vi "main.vi"(0 "Test Pins":T13, 1 "Caller Information":T10, 5 "Test Inputs":T7={"Load Current in A"=0.0, "Frequency in Hz"=[], "Input Voltage in V"=0.0, "FGen Peak-Peak Voltage in V"=1.0, "Resolution bandwidth in %"=1.0, "Sampling Rate multiplier"=10.0, "Take PSRR snapshot?"=TRUE, "Acquisition Time(s)"=0.2, "Horizontal Timing"=enum."Calculate Sampling Rate", "Advance Setting"={"Prepare"={"Load SMU Output Function"=enum."VoltageSource"}, "Stimulus and Measure"={"Loop Delay"=1, "Autoset Sampling Rate?"=TRUE, "Search Tolerance (+/- % of Freq.)"=5.0}}}, 11 "error in":errorcluster) -> (4 "Test Results":T14 {"Record Length in S" format="%#.5g"; "Sample Rate in S/s" format="%#.5g"; "PSRR in dB" format="%#.5g"; "Frequency in Hz" format="%#.5g"; "Detected Vin_ac_pp in V" format="%#.5g"; "Detected Vout_ac_pp in V" format="%#.5g"}, 15 "error out":errorcluster)   [LabVIEW 2020, in "LDO PSRR.lvlib"]
doc: "<b>Caller</b> Information is input for framework components. Mode should be set to <b>Automation</b> when running from TestStand. Sequence Context should be set to <b>ThisContext</b> when running from TestStand. The values will be updated everytime the setting is applied using \"Edit\" dialog.\n\n<b>Test Pins</b> is names of pins available in the pinmap file. Provide the right pins for the required functionality.\n\n<b>Test Inputs</b> is input required for the measurement to perform.\n\n<b>error in</b> is meant for the sequencing. <b>error in</b> should be <b>no error</b> always.\n\n<b>Test Results</b> contains all the measured data during the measurement and processed results.\n\n<b>error out</b> contains the error occured during measurement.\n\nCheck measurement documentation for more information (<Program Files>\\Soliton Technologies\\MeasurementSuite\\CodeModules\\LDO\\LDO PSRR.pdf)"
uses:
  LDO PSRR.lvlib
  Typedefs/Test Results.ctl
  Typedefs/Test Inputs.ctl
  Typedefs/Advance Test Input.ctl
  Reusables/Instrument APIs/Load Output Function.ctl
  <userlib>/_Soliton/Measurement Suite/Reusables/Plugin Common/Typedefs/Caller Events.ctl
  <userlib>/_Soliton/Measurement Suite/Reusables/Plugin Common/Typedefs/Caller Information.ctl
  <userlib>/_Soliton/Measurement Suite/Reusables/Plugin Common/Typedefs/Caller Mode.ctl
  Typedefs/Test Pins.ctl
  Typedefs/Pin Dropdown.ctl
  <userlib>/_Soliton/Measurement Suite/Reusables/Plugin Common/Typedefs/Termination Monitor Info.ctl
  <instrlib>/niFgen/niFgen.llb/niFgen Output Mode.ctl
  <instrlib>/niFgen/niFgen.llb/niFgen Waveform Type.ctl
  <vilib>/Utility/error.llb/DialogType.ctl
  ed717c1b-eec1-43b4-99c1-3d83852bef44.vi
  00c9e72c-dc14-40c2-acfc-7b2698a37ca7.vi
  d9360132-6dee-4b9e-876e-39170c807331.vi
  f5d431a0-41a8-4d91-8ed4-f3030fcb2f72.vi
  e32b1f2d-d2d3-47cf-a8ae-c4d1a59e525c.vi
  bb3e62c4-a2c2-4505-9438-f842dd651d6c.vi
  ce2ee1e5-697c-4608-b941-8c9b0f21ffd9.vi
  9f6bafd6-9b9c-4545-a9d9-e38da2077c76.vi
  c4032409-4502-45fd-bca3-2506d9579697.vi
  b2eee2bd-4b89-4e54-a034-5f4da275eb34.vi
  <userlib>/_Soliton/Measurement Suite/Reusables/InstrumentSessionAPIs/SessionManagerApiPath.vi
  <vilib>/Utility/sysdir.llb/Get System Directory.vi
  <vilib>/Utility/LVLibp/Get Exported File Path.vi
  <userlib>/_Soliton/Measurement Suite/Reusables/Errors/Error 6001.vi
  <userlib>/_Soliton/Measurement Suite/Reusables/Plugin Common/Plugin Common.lvlib
  <userlib>/_Soliton/Measurement Suite/Reusables/Queue Driver/Plugin Queue Driver.lvlib
panel:
  out "Progress":i32(slide) scale=-1.0..5.0
  in  "Terminate":bool
  in  "Run":bool caption="Measure"
  in  "Exit":bool
  out "Header":string
  in  "Tab Enum":T1(radio)
  out "Tab Control":T2(tab)
  in  "SystemSetup":T4={"Set Input Voltage"={"PinStatus"=0, "PinName"="", "Info"=TRUE}, "Set Frequency"={"PinStatus"=0, "PinName"="", "Info"=TRUE}, "Set Load Current"={"PinStatus"=0, "PinName"="", "Info"=TRUE}, "Measure Input Voltage"={"PinStatus"=0, "PinName"="", "Info"=TRUE}, "Measure Output Voltage"={"PinStatus"=0, "PinName"="", "Info"=TRUE}}
  in  "Sampling Rate Multiplier":dbl=10.0 min=2.0 max=100.0 format="%#_6p"
  in  "Minimum Resolution Bandwidth (%)":dbl=1.0 min=0.001 max=100.0 format="%#_6f"
  in  "Step Input":T5={"Minimum Frequency (Hz)"=10.0, "Maximum Frequency (Hz)"=10000000.0} {"Maximum Frequency (Hz)" min=10.0 max=80000000.0 format="%#_6p"; "Minimum Frequency (Hz)" items=["10Hz"=10.0, "100Hz"=100.0, "1kHz"=1000.0, "100kHz"=100000.0]}
  in  "Customize Sweep Value":bool
  in  "Input Voltage (V)":dbl format="%#_6p"
  in  "Load Current (A)":dbl format="%#_6p"
  in  "Advanced Settings":bool
  in  "Pk-Pk Voltage (V)":dbl=1.0 caption="FGen Peak-Peak Voltage (V)" format="%#_6p"
  in  "Frequency (Hz)":dbl[](array[numeric]) format="%#_6p"
  out "Result Tab":T6(tab)
  out "Frequency Vs PSRR":cluster{"Iload (mA)":dbl[], "Vout (V)":dbl[]}(graph)
  in  "Take PSRR snapshot?":bool=TRUE
  out "Measured Values":string[][](table)
  in  "Result Enum":T6(radio)
  in  "ErrorOccured":errorcluster
  in  "Caller Events":T12
  in  "DataLogPath":path
  # "Supports NIScopeInstrument"
  # "Supports NIScopeInstrument"
  # "Supports NIFGenInstrument"
  # "Supports NIDCPowerInstrument"
  # "Supports NIDCPowerInstrument"
  # "SMU Settings"
  # "FGen Settings"
  # "Fill Frequency using the following"
  # "Oscilloscope Settings"
  # "Resolution Bandwidth (%) is the percentage of minimum separation required between two frequency\nMinimum Sampling Rate = Frequency * Sampling Rate Multiplier"
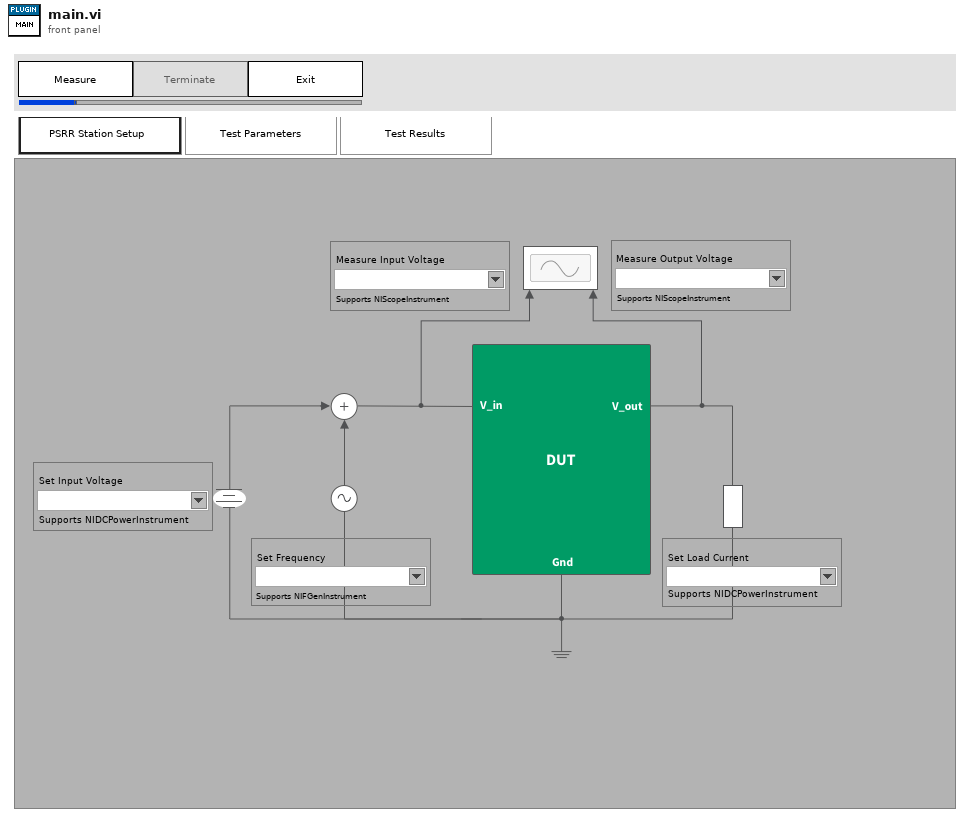
[diagram p1: front panel]
types:
  T1 = enum32{"Station Setup", "Test Parameters", "Test Results"}
  T2 = enum32{"Station Setup", "Test Parameters", "Test Results", "Debug"}
  T3 = typedef "LDO PSRR.lvlib/Pin Dropdown.ctl" = cluster{"PinStatus":u16, "PinName":string, "Info":bool}
  T4 = cluster{"Set Input Voltage":T3, "Set Frequency":T3, "Set Load Current":T3, "Measure Input Voltage":T3, "Measure Output Voltage":T3}
  T5 = cluster{"Minimum Frequency (Hz)":dbl, "Maximum Frequency (Hz)":dbl}
  T6 = enum32{"Line Regulation Curve", "Measured Value Table View"}
  T7 = typedef "LDO PSRR.lvlib/Test Inputs.ctl" = cluster{"Load Current in A":dbl, "Frequency in Hz":dbl[], "Input Voltage in V":dbl, "FGen Peak-Peak Voltage in V":dbl, "Resolution bandwidth in %":dbl, "Sampling Rate multiplier":dbl, "Take PSRR snapshot?":bool, "Acquisition Time(s)":dbl, "Horizontal Timing":enum32{"Calculate Sampling Rate", "Calculate Acquisition Time", "Calculate Record Length"}, "Advance Setting":T8}
  T8 = typedef "LDO PSRR.lvlib/Advance Test Input.ctl" = cluster{"Prepare":cluster{"Load SMU Output Function":T9}, "Stimulus and Measure":cluster{"Loop Delay":u32, "Autoset Sampling Rate?":bool, "Search Tolerance (+/- % of Freq.)":dbl}}
  T9 = typedef "Load Output Function.ctl" = enum16{"VoltageSource", "CurrentSource"}
  T10 = typedef "Plugin Common.lvlib/Caller Information.ctl" = cluster{"Mode":T11, "Sequence Context":refnum<k7>}
  T11 = typedef "Plugin Common.lvlib/Caller Mode.ctl" = enum16{"Standalone", "Automation", "MeasurementSuite"}
  T12 = typedef "Plugin Common.lvlib/Caller Events.ctl" = cluster{"Caller Event":refnum<user-event>}
  T13 = typedef "LDO PSRR.lvlib/Test Pins.ctl" = cluster{"Set Input Voltage":string, "Measure Input Voltage":string, "Set Load Current":string, "Measure Output Voltage":string, "Set Frequency":string}
  T14 = typedef "LDO PSRR.lvlib/Test Results.ctl" = cluster{"Frequency in Hz":dbl[], "Detected Vin_ac_pp in V":dbl[], "Detected Vout_ac_pp in V":dbl[], "PSRR in dB":dbl[], "Sample Rate in S/s":dbl[], "Record Length in S":dbl[]}
  T15 = typedef "Plugin Common.lvlib/Termination Monitor Info.ctl" = cluster{"Caller Information":T10, "Execution":refnum<k7>, "Termination Monitor":refnum<k7>, "Type":string, "Plugin Name":string}
  T16 = cluster{"Termination Monitor Info":T15, "Test Inputs":T7, "Test Results":T14, "Test Results[][]":string[][], "Test Pins":T13, "Logger Folder Path":path, "Scope Channels":string, "Valid Logger path?":bool, "Logger file path":path, "UI Ctls":refnum<vi>[], "Minimum Sampling Rate (S/s)":dbl, "Minimum Record Length (S)":i32}
  T17 = enum8{"Enabled", "Disabled", "Disabled and Grayed Out"}
  T18 = cluster{"Set Vin":T3, "Set Frequency":T3, "Set Iload":T3, "Measure Vin":T3, "Measure Vout":T3}
  T19 = cluster{"Minimum Frequency (Hz)":dbl, "Maximum Frequency Hz)":dbl}
  T20 = typedef "niFgen Waveform Type.ctl" = i32
  T21 = typedef "niFgen Output Mode.ctl" = u32
  T22 = cluster{"relativeInitialX":dbl, "xIncrement":dbl, "wfm":dbl[]}
  T23 = cluster{"Frequency in Hz":dbl[], "PSRR in dB":dbl[]}
  T24 = typedef "DialogType.ctl" = u16
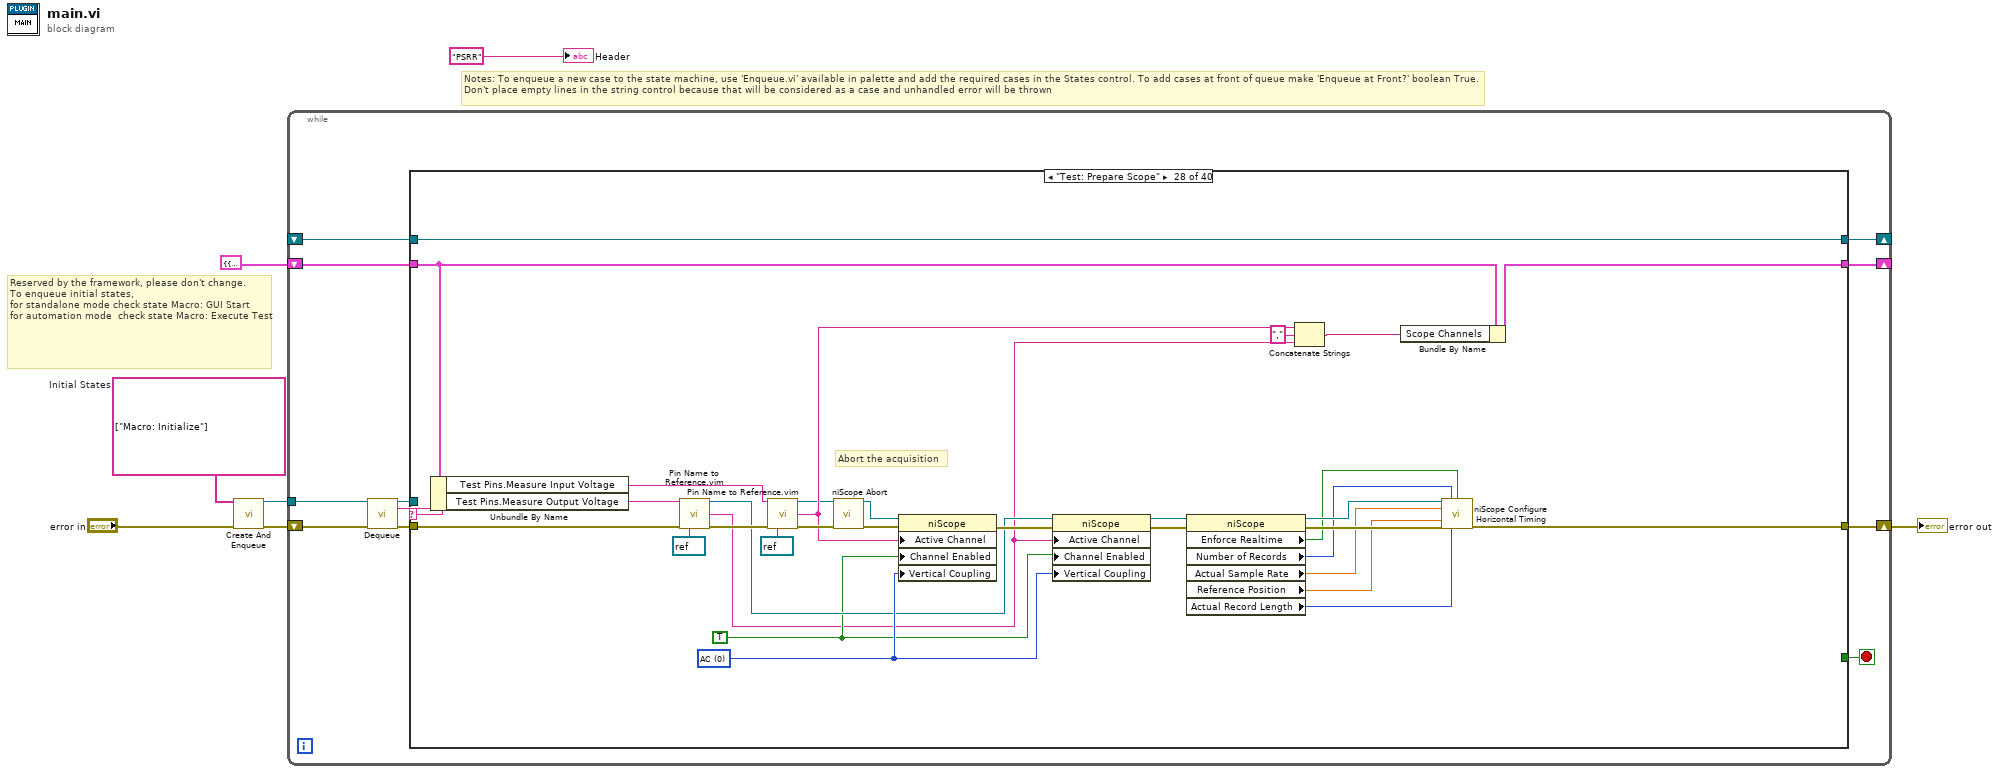
[diagram p0: block diagram]
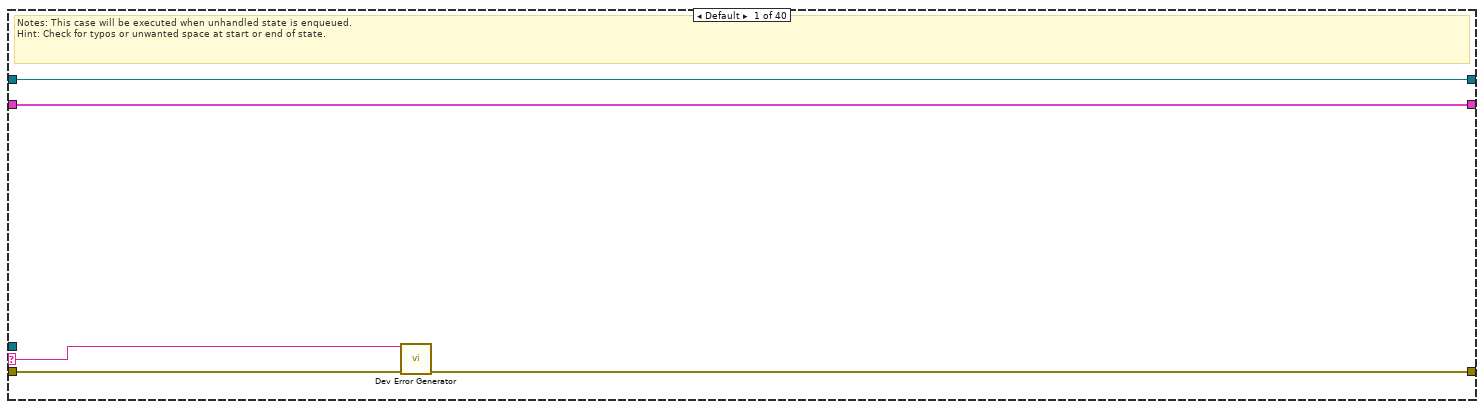
[diagram p2: hidden frame]
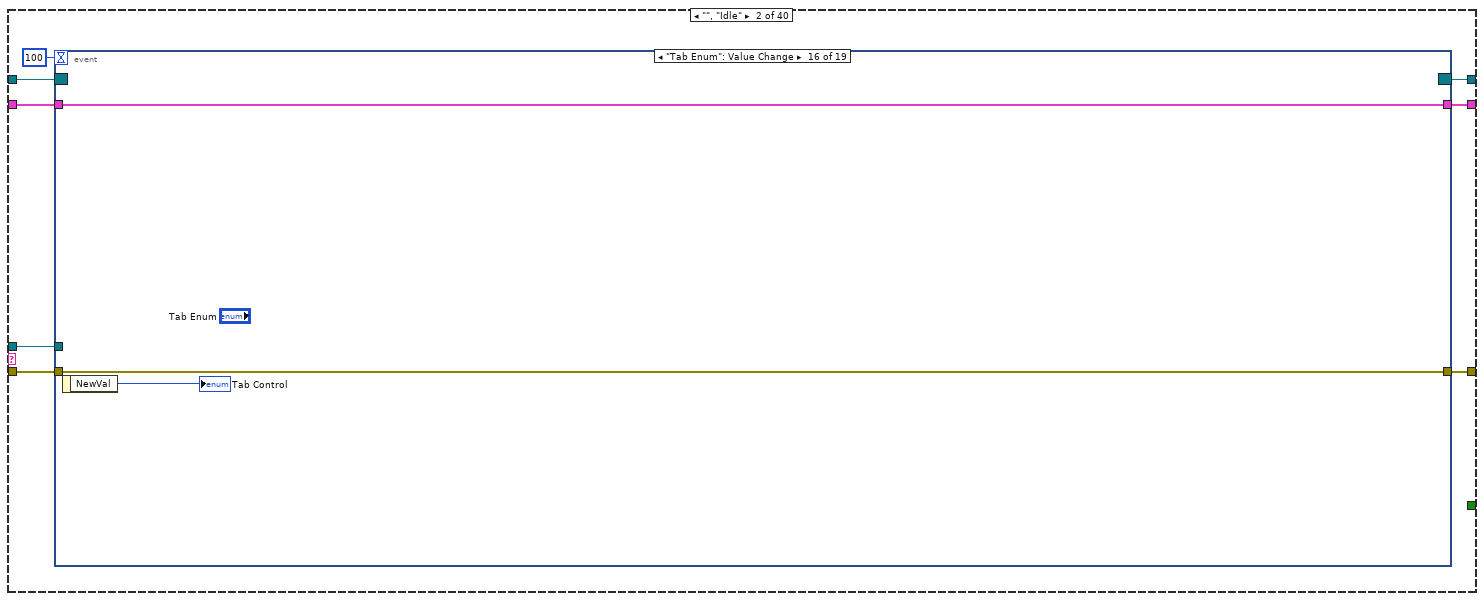
[diagram p3: hidden frame]
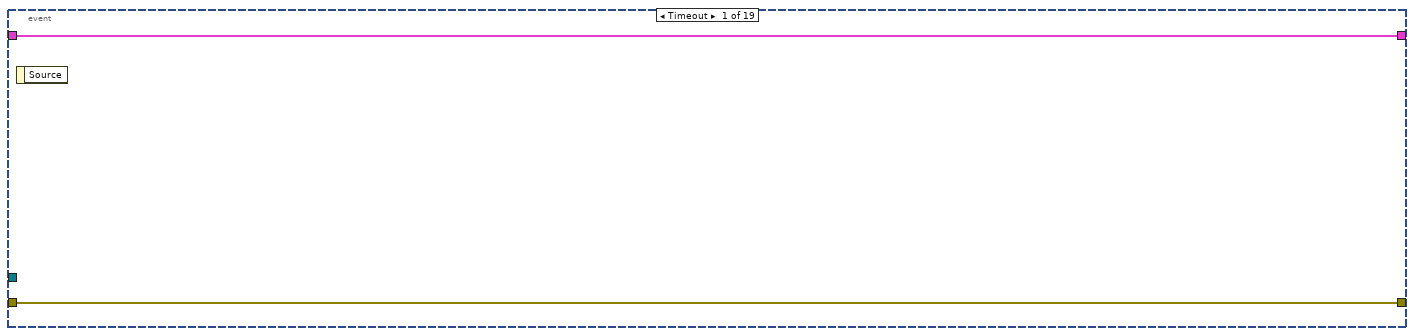
[diagram p4: hidden frame]
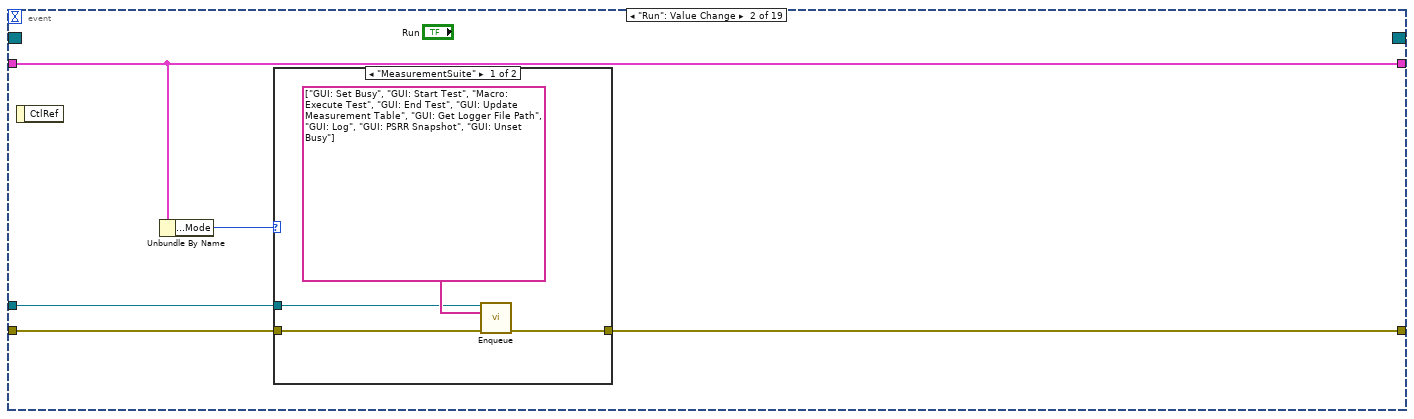
[diagram p5: hidden frame]
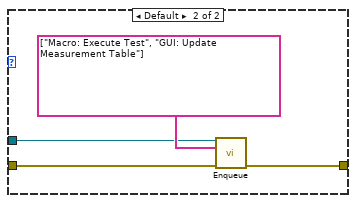
[diagram p6: hidden frame]
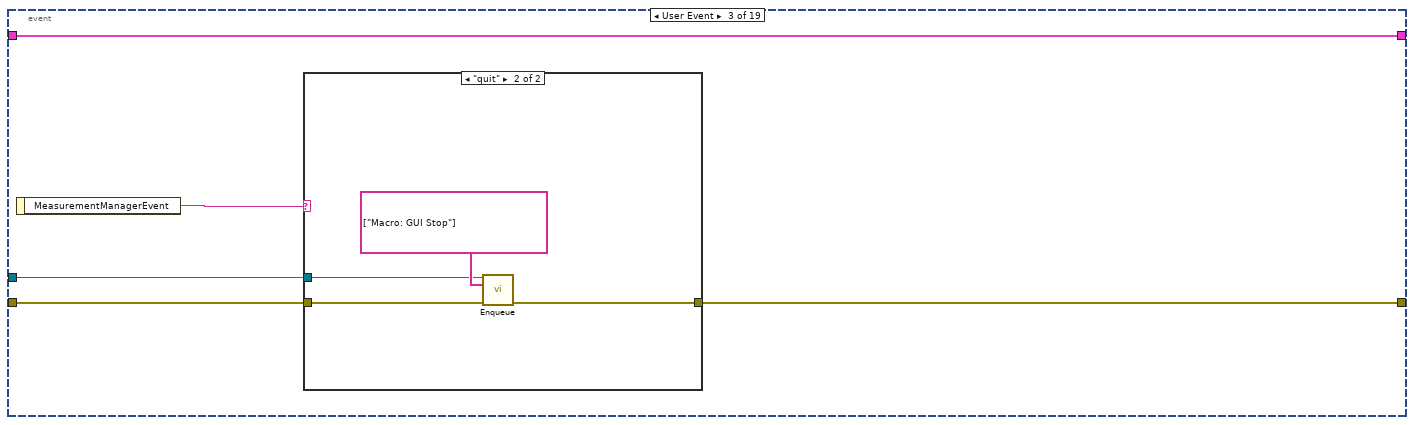
[diagram p7: hidden frame]
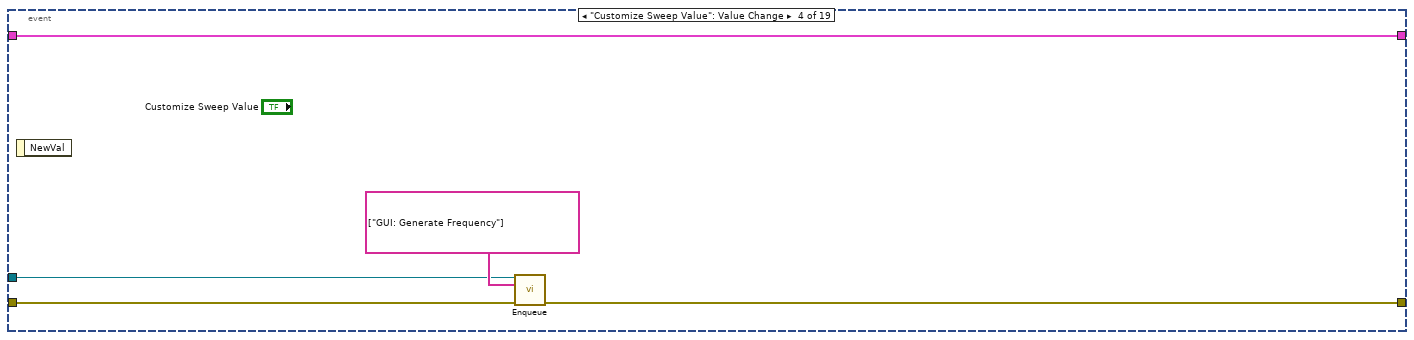
[diagram p9: hidden frame]
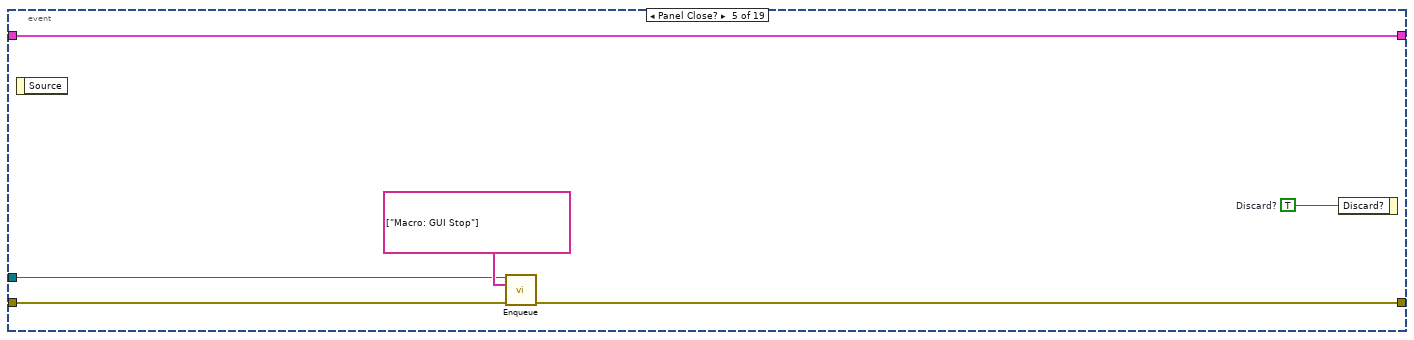
[diagram p10: hidden frame]
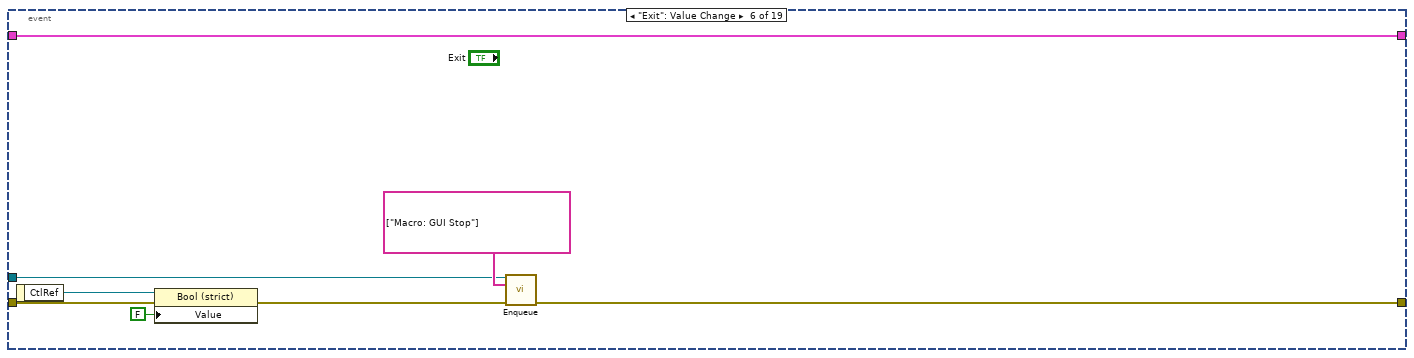
[diagram p11: hidden frame]
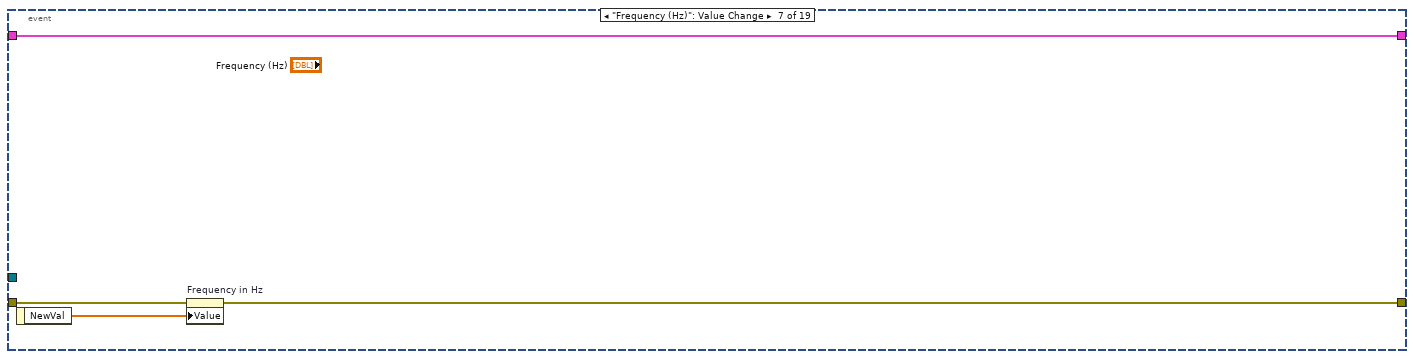
[diagram p12: hidden frame]
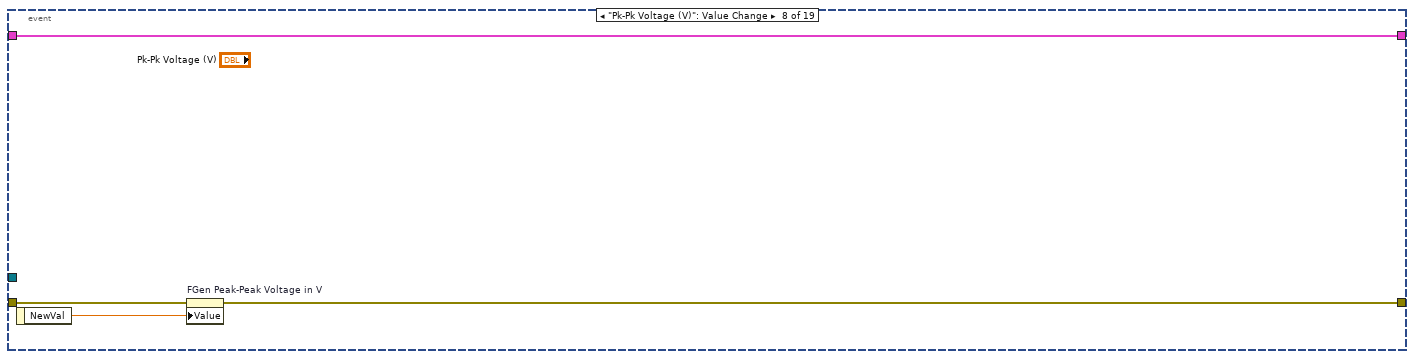
[diagram p13: hidden frame]
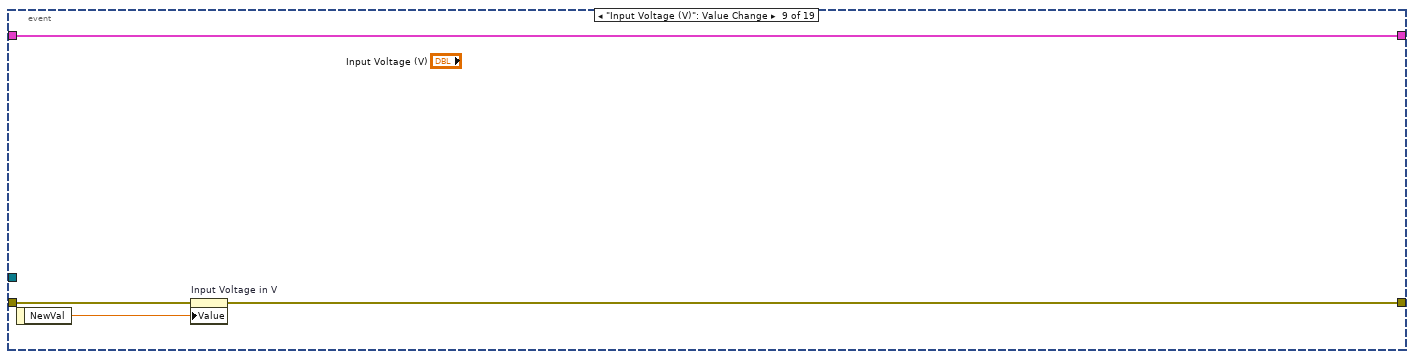
[diagram p14: hidden frame]
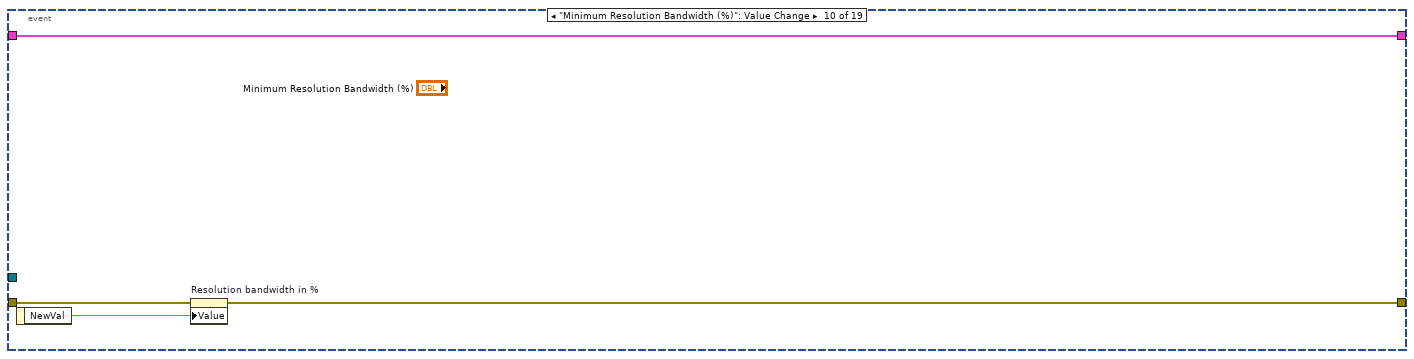
[diagram p15: hidden frame]
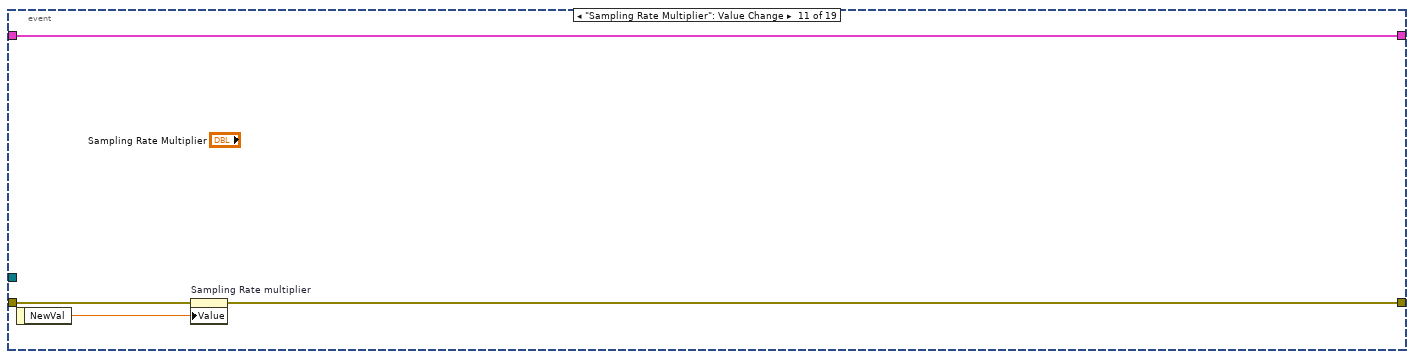
[diagram p16: hidden frame]
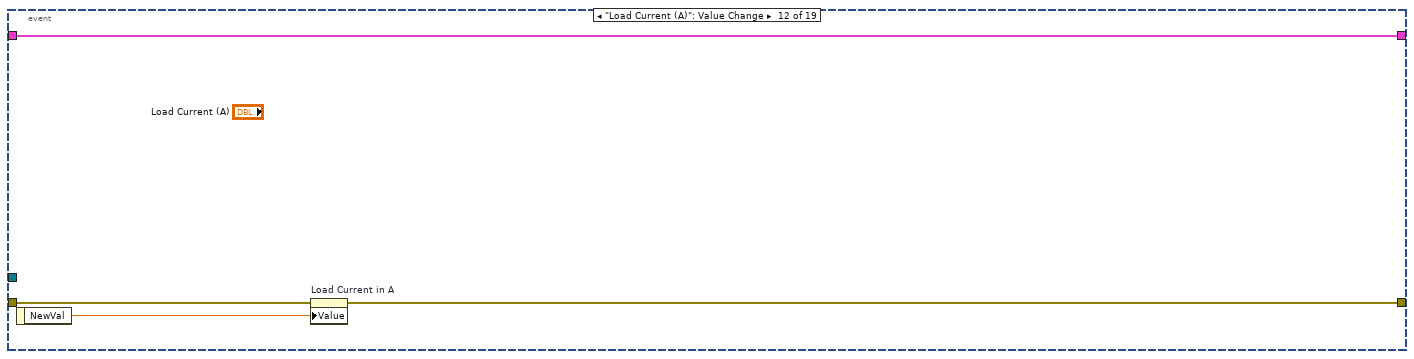
[diagram p17: hidden frame]
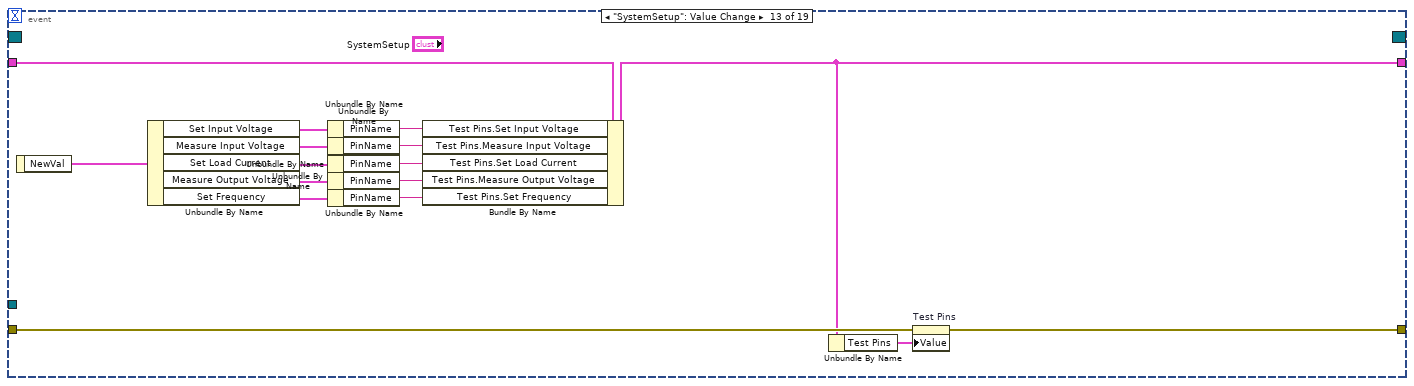
[diagram p18: hidden frame]
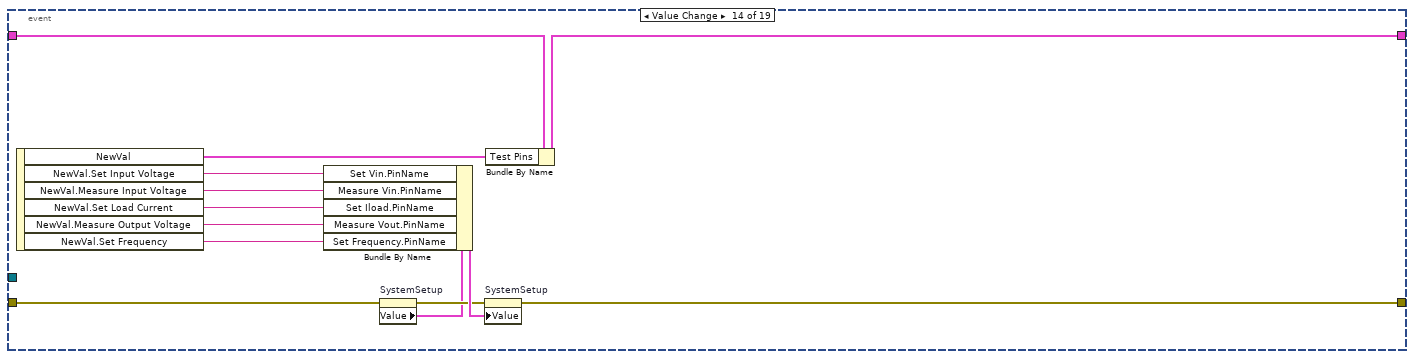
[diagram p19: hidden frame]
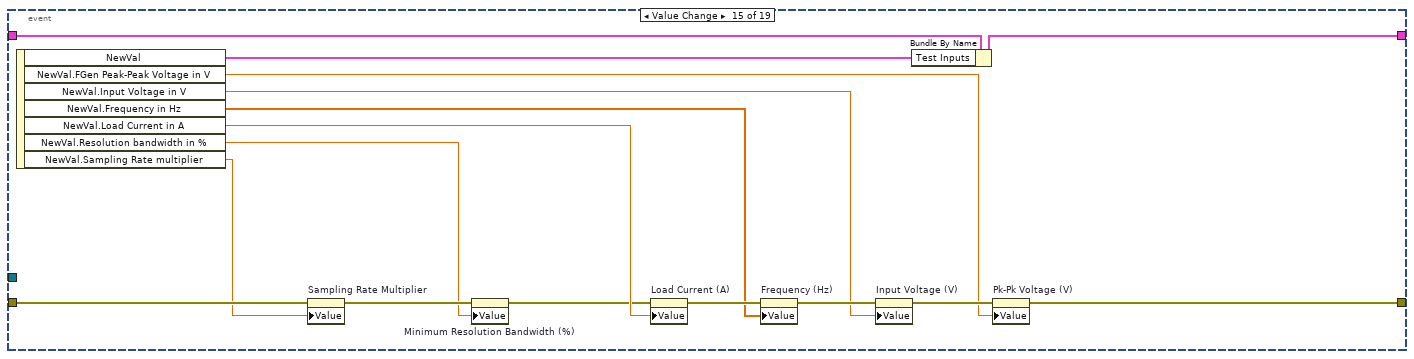
[diagram p20: hidden frame]
diagram:
  w7 = string[] ["Macro: Initialize"]  # Initial States
  # "Notes: To enqueue a new case to the state machine, use 'Enqueue.vi' available in palette and add the required cases in the States control. To add cases at front of queue make 'Enqueue at Front?' boolean True. Don't place empty lines in the string control because that will be considered as a case and unhandled error will be thrown"
  # "Reserved by the framework, please don't change. \nTo enqueue initial states,\nfor standalone mode check state Macro: GUI Start\nfor automation mode  check state Macro: Execute Test"
  n1 = call <userlib>:"Create And Enqueue.vi"("Initial States"=w7, "error in (no error)"="error in") -> ("Queue out"=w5:refnum<queue>, "error out"=w3:errorcluster)  [unwired: 12 in]
  n2 = while {
    shift-right: [w18] -> w4
    shift-left: w3 -> [w16]
    shift-right: [w14] -> _
    shift-left: T16 {"Termination Monitor Info"={"Caller Information"={"Mode"=enum."Standalone", "Sequence Context"=refnum}, "Execution"=refnum, "Termination Monitor"=refnum, "Type"="", "Plugin Name"=""}, "Test Inputs"={"Load Current in A"=0.0, "Frequency in Hz"=[], "Input Voltage in V"=0.0, "FGen Peak-Peak Voltage in V"=0.0, "Resolution bandwidth in %"=20000000.0, "Sampling Rate multiplier"=1000.0, "Take PSRR snapshot?"=FALSE, "Acquisition Time(s)"=0.0, "Horizontal Timing"=enum."Calculate Sampling Rate", "Advance Setting"={"Prepare"={"Load SMU Output Function"=enum."VoltageSource"}, "Stimulus and Measure"={"Loop Delay"=0, "Autoset Sampling Rate?"=TRUE, "Search Tolerance (+/- % of Freq.)"=0.0}}}, "Test Results"={"Frequency in Hz"=[], "Detected Vin_ac_pp in V"=[], "Detected Vout_ac_pp in V"=[], "PSRR in dB"=[], "Sample Rate in S/s"=[], "Record Length in S"=[]}, "Test Results[][]"=[], "Test Pins"={"Set Input Voltage"="", "Measure Input Voltage"="", "Set Load Current"="", "Measure Output Voltage"="", "Set Frequency"=""}, "Logger Folder Path"=path "", "Scope Channels"="", "Valid Logger path?"=FALSE, "Logger file path"=path "", "UI Ctls"=[], "Minimum Sampling Rate (S/s)"=0.0, "Minimum Record Length (S)"=0} -> [w13]
    tunnel: w5 -> [w12]
    shift-right: [w9] -> _
    shift-left: _ -> [w10]
    stop <- w17 stop-if-true
    n3 = call <userlib>:"Dequeue.vi"("Queue in"=w12, "error in (no error)"=w16) -> ("Queue out"=w11:refnum<queue>, "Dequeued State"=w8:string, "error out"=w15:errorcluster)  [unwired: 11 in]
    n4 = case shown="\"Test: Prepare Scope\"" w8 {
      selector: w8 -> [w21 _ _ _ _ _ _ _ _ _ _ _ _ _ _ _ _ _ _ _ _ _ _ _ _ _ _ _ _ _ _ _ _ _ _ _ _ _ _ _]
      tunnel: w15 -> [w20 w28 w164 w173 w182 w189 w196 w201 w228 w239 w243 w246 w257 w272 w277 w290 w306 w321 w345 w359 w376 w386 w391 w398 w403 w417 w427 w459 w466 w473 w497 w595 w606 w624 w636 w638 w650 w658 w665 w683]
      tunnel: [w22 w29 w164 w176 w183 w190 w197 w201 w226 w237 w241 w246 w251 w272 w276 w289 w307 w319 w346 w360 w377 w386 w392 w399 w403 w411 w424 w458 w464 w471 w499 w580 w599 w612 w636 w638 w647 w658 w663 w677] -> w18
      tunnel: [_ _ _ _ _ _ _ _ _ _ _ _ _ _ _ _ _ _ _ _ _ _ _ _ _ _ _ _ _ _ _ _ _ _ _ _ _ _ w660 TRUE] -> w17
      tunnel: [w23 w31 w163 w166 w184 w191 w198 w200 w217 w238 w242 w245 w249 w266 w278 w291 w304 w316 w347 w361 w383 w385 w390 w397 w402 w410 w429 w457 w465 w472 w501 w597 w608 w626 w635 w644 w655 w657 w662 w684] -> w14
      tunnel: w13 -> [w23 w30 w163 w177 w184 w191 w198 w200 w233 w238 w242 w245 w248 w265 w278 w291 w304 w315 w347 w361 w383 w385 w389 w396 w402 w420 w429 w456 w465 w472 w502 w597 w608 w626 w634 w644 w655 w657 w662 w684]
      tunnel: w11 -> [_ w24 _ w175 w180 w187 w194 _ _ _ _ _ _ _ _ _ _ _ _ _ _ _ _ _ _ _ _ _ _ _ _ _ _ _ _ _ _ _ w659 w682]
      tunnel: w10 -> [w19 w26 w162 w174 w179 w186 w193 w199 w232 _ w240 w244 w258 w271 w284 w297 w313 w322 w348 w362 w382 w384 w393 w400 w401 w419 w430 w461 w467 w474 w500 w598 w609 w627 w637 w643 w654 w656 w664 w681]
      tunnel: [w19 w25 w162 w174 w179 w186 w193 w199 w232 w236 w240 w244 w258 w271 w284 w297 w313 w322 w348 w362 w382 w384 w393 w400 w401 w419 w430 w461 w467 w474 w500 w598 w609 w627 w637 w643 w654 w656 w664 w681] -> w9
      frame Default {
        # "Notes: This case will be executed when unhandled state is enqueued. \nHint: Check for typos or unwanted space at start or end of state."
        n5 = call <userlib>:"Dev Error Generator.vi"("State"=w21, "error in (no error)"=w20) -> ("error out"=w22:errorcluster)  [unwired: 13 in]
      }
      frame "", "Idle" {
        n6 = event shown="[15] \"Tab Enum\": Value Change" {
          selector: w26 -> [_ _ _ _ _ _ _ _ _ _ _ _ _ _ _ _ _ _ _]
          dyn-events: [_ _ _ _ _ _ _ _ _ _ _ _ _ _ _ _ _ _ _] -> w25
          timeout: 100 -> [_ _ _ _ _ _ _ _ _ _ _ _ _ _ _ _ _ _ _]
          tunnel: [w33 w35 w51 w61 w67 w75 w76 w81 w87 w91 w95 w99 w101 w126 w140 w147 w150 w154 w160] -> w31
          tunnel: w30 -> [w33 w35 w51 w61 w67 w75 w76 w81 w87 w91 w95 w99 w105 w125 w139 w147 w150 w154 w159]
          tunnel: [w32 w38 w49 w59 w64 w73 w78 w82 w86 w90 w94 w98 w103 w127 w142 w146 w149 w152 w156] -> w29
          tunnel: w28 -> [w32 w37 w50 w58 w63 w72 w79 w83 w85 w89 w93 w97 w102 w128 w133 w146 w149 w153 w161]
          tunnel: w24 -> [_ w36 w47 w57 w62 w71 _ _ _ _ _ _ _ _ _ _ _ _ _]
          event Timeout {
            n7 = event-data() -> ()  [unwired: 1 in, 1 out]
          }
          event "Run": Value Change {
            n8 = event-data() -> ()  [unwired: 1 in, 1 out]
            n9 = Unbundle By Name(w35) -> ("Termination Monitor Info.Caller Information.Mode"=w34:T11)
            n10 = case shown="\"MeasurementSuite\"" w34 {
              tunnel: [w41 w45] -> w38
              tunnel: w37 -> [w40 w44]
              tunnel: w36 -> [w39 w43]
              frame "MeasurementSuite" {
                n11 = call <userlib>:"Enqueue.vi"("Queue in"=w39, "States"=string[] ["GUI: Set Busy", "GUI: Start Test", "Macro: Execute Test", "GUI: End Test", "GUI: Update Measurement Table", "GUI: Get Logger File Path", "GUI: Log", "GUI: PSRR Snapshot", "GUI: Unset Busy"], "error in (no error)"=w40) -> ("error out"=w41:errorcluster)  [unwired: 11 in, 1 out]
              }
              frame Default {
                n12 = call <userlib>:"Enqueue.vi"("Queue in"=w43, "States"=string[] ["Macro: Execute Test", "GUI: Update Measurement Table"], "error in (no error)"=w44) -> ("error out"=w45:errorcluster)  [unwired: 11 in, 1 out]
              }
            }
          }
          event User Event {
            n13 = event-data() -> ("MeasurementManagerEvent"=w48:string)  [unwired: 1 in]
            n14 = case shown="\"quit\"" w48 {
              tunnel: [w52 w53] -> w49
              tunnel: w50 -> [w52 w55]
              tunnel: w47 -> [_ w54]
              frame Default {
              }
              frame "quit" {
                n15 = call <userlib>:"Enqueue.vi"("Queue in"=w54, "States"=string[] ["Macro: GUI Stop"], "error in (no error)"=w55) -> ("error out"=w53:errorcluster)  [unwired: 11 in, 1 out]
              }
            }
          }
          event "Customize Sweep Value": Value Change {
            n16 = event-data() -> ()  [unwired: 1 in, 1 out]
            n17 = call <userlib>:"Enqueue.vi"("Queue in"=w57, "States"=string[] ["GUI: Generate Frequency"], "error in (no error)"=w58) -> ("error out"=w59:errorcluster)  [unwired: 11 in, 1 out]
          }
          event Panel Close? {
            w66 = TRUE  # Discard?
            n18 = event-data() -> ()  [unwired: 1 in, 1 out]
            n19 = call <userlib>:"Enqueue.vi"("Queue in"=w62, "States"=string[] ["Macro: GUI Stop"], "error in (no error)"=w63) -> ("error out"=w64:errorcluster)  [unwired: 11 in, 1 out]
            n20 = event-data("Discard?"=w66) -> ()  [unwired: 1 in, 1 out]
          }
          event "Exit": Value Change {
            n21 = event-data() -> ("CtlRef"=w69:refnum<vi>)  [unwired: 1 in]
            n22 = property class="Bool (strict)"(reference=w69, error in=w72, "Value"=FALSE) -> (error out=w70:errorcluster)  [unwired: 1 out]
            n23 = call <userlib>:"Enqueue.vi"("Queue in"=w71, "States"=string[] ["Macro: GUI Stop"], "error in (no error)"=w70) -> ("error out"=w73:errorcluster)  [unwired: 11 in, 1 out]
          }
          event "Frequency (Hz)": Value Change {
            n24 = event-data() -> ("NewVal"=w77:dbl[])  [unwired: 1 in]
            n25 = property on="Frequency in Hz" class="Arr (strict)"(error in=w79, "Value"=w77) -> (error out=w78:errorcluster)  [unwired: 1 in, 1 out]
          }
          event "Pk-Pk Voltage (V)": Value Change {
            n26 = event-data() -> ("NewVal"=w80:dbl)  [unwired: 1 in]
            n27 = property on="FGen Peak-Peak Voltage in V" class="DigNum (strict)"(error in=w83, "Value"=w80) -> (error out=w82:errorcluster)  [unwired: 1 in, 1 out]
          }
          event "Input Voltage (V)": Value Change {
            n28 = event-data() -> ("NewVal"=w84:dbl)  [unwired: 1 in]
            n29 = property on="Input Voltage in V" class="DigNum (strict)"(error in=w85, "Value"=w84) -> (error out=w86:errorcluster)  [unwired: 1 in, 1 out]
          }
          event "Minimum Resolution Bandwidth (%)": Value Change {
            n30 = event-data() -> ("NewVal"=w88:dbl)  [unwired: 1 in]
            n31 = property on="Resolution bandwidth in %" class="DigNum (strict)"(error in=w89, "Value"=w88) -> (error out=w90:errorcluster)  [unwired: 1 in, 1 out]
          }
          event "Sampling Rate Multiplier": Value Change {
            n32 = event-data() -> ("NewVal"=w92:dbl)  [unwired: 1 in]
            n33 = property on="Sampling Rate multiplier" class="DigNum (strict)"(error in=w93, "Value"=w92) -> (error out=w94:errorcluster)  [unwired: 1 in, 1 out]
          }
          event "Load Current (A)": Value Change {
            n34 = event-data() -> ("NewVal"=w96:dbl)  [unwired: 1 in]
            n35 = property on="Load Current in A" class="DigNum (strict)"(error in=w97, "Value"=w96) -> (error out=w98:errorcluster)  [unwired: 1 in, 1 out]
          }
          event "SystemSetup": Value Change {
            n36 = event-data() -> ("NewVal"=w104:T4)  [unwired: 1 in]
            n37 = Unbundle By Name(w104) -> ("Set Input Voltage"=w110:T3, "Measure Input Voltage"=w109:T3, "Set Load Current"=w108:T3, "Measure Output Voltage"=w107:T3, "Set Frequency"=w106:T3)
            n38 = Unbundle By Name(w110) -> ("PinName"=w115:string)
            n39 = Unbundle By Name(w109) -> ("PinName"=w114:string)
            n40 = Unbundle By Name(w108) -> ("PinName"=w113:string)
            n41 = Unbundle By Name(w107) -> ("PinName"=w112:string)
            n42 = Unbundle By Name(w106) -> ("PinName"=w111:string)
            n43 = Bundle By Name(cluster=w105, "Test Pins.Set Input Voltage"=w115, "Test Pins.Measure Input Voltage"=w114, "Test Pins.Set Load Current"=w113, "Test Pins.Measure Output Voltage"=w112, "Test Pins.Set Frequency"=w111) -> (w101:T16)
            n44 = Unbundle By Name(w101) -> ("Test Pins"=w100:T13)
            n45 = property on="Test Pins" class="Clust (strict)"(error in=w102, "Value"=w100) -> (error out=w103:errorcluster)  [unwired: 1 in, 1 out]
          }
          event Value Change {
            n46 = event-data() -> ("NewVal"=w116:T13, "NewVal.Set Input Voltage"=w124:string, "NewVal.Measure Input Voltage"=w123:string, "NewVal.Set Load Current"=w122:string, "NewVal.Measure Output Voltage"=w121:string, "NewVal.Set Frequency"=w117:string)  [unwired: 1 in]
            n47 = property on="SystemSetup" class="Clust (strict)"(error in=w128) -> (error out=w119:errorcluster, "Value"=w118:T18)  [unwired: 1 in, 1 out]
            n48 = Bundle By Name(cluster=w118, "Set Vin.PinName"=w124, "Measure Vin.PinName"=w123, "Set Iload.PinName"=w122, "Measure Vout.PinName"=w121, "Set Frequency.PinName"=w117) -> (w120:T18)
            n49 = property on="SystemSetup" class="Clust (strict)"(error in=w119, "Value"=w120) -> (error out=w127:errorcluster)  [unwired: 1 in, 1 out]
            n50 = Bundle By Name(cluster=w125, "Test Pins"=w116) -> (w126:T16)
          }
          event Value Change {
            n51 = event-data() -> ("NewVal"=w134:T7, "NewVal.FGen Peak-Peak Voltage in V"=w135:dbl, "NewVal.Input Voltage in V"=w136:dbl, "NewVal.Frequency in Hz"=w137:dbl[], "NewVal.Load Current in A"=w138:dbl, "NewVal.Resolution bandwidth in %"=w130:dbl, "NewVal.Sampling Rate multiplier"=w129:dbl)  [unwired: 1 in]
            n52 = property on="Sampling Rate Multiplier" class="DigNum (strict)"(error in=w133, "Value"=w129) -> (error out=w131:errorcluster)  [unwired: 1 in, 1 out]
            n53 = property on="Minimum Resolution Bandwidth (%)" class="DigNum (strict)"(error in=w131, "Value"=w130) -> (error out=w132:errorcluster)  [unwired: 1 in, 1 out]
            n54 = property on="Load Current (A)" class="DigNum (strict)"(error in=w132, "Value"=w138) -> (error out=w141:errorcluster)  [unwired: 1 in, 1 out]
            n55 = property on="Frequency (Hz)" class="Arr (strict)"(error in=w141, "Value"=w137) -> (error out=w144:errorcluster)  [unwired: 1 in, 1 out]
            n56 = property on="Input Voltage (V)" class="DigNum (strict)"(error in=w144, "Value"=w136) -> (error out=w143:errorcluster)  [unwired: 1 in, 1 out]
            n57 = Bundle By Name(cluster=w139, "Test Inputs"=w134) -> (w140:T16)
            n58 = property on="Pk-Pk Voltage (V)" class="DigNum (strict)"(error in=w143, "Value"=w135) -> (error out=w142:errorcluster)  [unwired: 1 in, 1 out]
          }
          event "Tab Enum": Value Change {
            n59 = event-data() -> ("NewVal"=→"Tab Control":T1)  [unwired: 1 in]
          }
          event "Result Enum": Value Change {
            n60 = event-data() -> ("NewVal"=→"Result Tab":T6)  [unwired: 1 in]
          }
          event "Take PSRR snapshot?": Value Change {
            n61 = event-data() -> ("NewVal"=w151:bool)  [unwired: 1 in]
            n62 = property on="Take PSRR snapshot?" class="Bool (strict)"(error in=w153, "Value"=w151) -> (error out=w152:errorcluster)  [unwired: 1 in, 1 out]
          }
          event "Advanced Settings": Value Change {
            n63 = event-data() -> ()  [unwired: 1 in, 1 out]
            n64 = Unbundle By Name(w159) -> ("Test Inputs.Advance Setting"=w158:T8)
            n65 = call "Advance Settings UI.vi"("Advance Setting"=w158, "error in (no error)"=w161) -> ("Advance Setting Out"=w155:T8, "error out"=w157:errorcluster)  [unwired: 12 in]
            n66 = Bundle By Name(cluster=w159, "Test Inputs.Advance Setting"=w155) -> (w160:T16)
            n67 = property on="Advance Setting" class="Clust (strict)"(error in=w157, "Value"=w155) -> (error out=w156:errorcluster)  [unwired: 1 in, 1 out]
          }
        }
      }
      frame "----------------- Macro ---------------" {
        # "Not used. category splitter"
      }
      frame "Macro: Initialize" {
        w170 = string[] ["Macro: GUI Start"]  # Standalone: Start the debug
        w171 = string[] ["Macro: Execute Test", "Exit"]  # Automation: Execute and stop
        # "Hidden in UI"
        # "This case decides the mode of the execution. Debug Mode: The plugin will act as a standalone GUI where user can change inputs, run test and debug the system. automation mode: The plugin will act as a flat code and go through all the test procedures and stops."
        n68 = call <userlib>:"Get Mode.vi"("Caller Information"="Caller Information", "error in (no error)"=w173) -> ("Automation(F) \\ Standalone (T)"=w169:bool, "error out"=w172:errorcluster)  [unwired: 12 in]
        n69 = Bundle By Name(cluster=w177, "Termination Monitor Info.Caller Information"="Caller Information") -> (w166:T16)
        n70 = Select(t=w170, s=w169, f=w171) -> (s? t:f=w168:string[])
        n71 = call <userlib>:"Enqueue.vi"("Queue in"=w175, "States"=w168, "Enqueue at Front?(F)"=TRUE, "error in (no error)"=w172) -> ("error out"=w176:errorcluster)  [unwired: 10 in, 1 out]
      }
      frame "Macro: Execute Test" {
        w181 = string[] ["TerminationMonitor: Start", "Test: Start", "Test: Prepare DCPower", "Test: Prepare Scope", "Test: Set Input Voltage", "Test: Set Load Current", "Test: Sweep Over Frequency", "Test: Cleanup DCPower", "Test: Cleanup Fgen", "Test: Cleanup Scope", "Test: Calculate PSRR", "Test: Update UI", "Test: End", "TerminationMonitor: Stop"]  # Test Procedure
        # "List the states required for the test procedure. This state will be called in both automation mode and standalone mode when requested to run the test.\nDont remove 'Test: Start' and 'Test: End'."
        n72 = call <userlib>:"Enqueue.vi"("Queue in"=w180, "States"=w181, "Enqueue at Front?(F)"=TRUE, "error in (no error)"=w182) -> ("error out"=w183:errorcluster)  [unwired: 10 in, 1 out]
      }
      frame "Macro: GUI Start" {
        # "Initialize the data cluster for the standalone mode and register for the event from caller.\nDon't remove 'GUI: Initialize Data' and 'GUI: Register Event'."
        n73 = call <userlib>:"Enqueue.vi"("Queue in"=w187, "States"=string[] ["GUI: Initialize Data", "GUI: Register Event"], "Enqueue at Front?(F)"=TRUE, "error in (no error)"=w189) -> ("error out"=w190:errorcluster)  [unwired: 10 in, 1 out]
      }
      frame "Macro: GUI Stop" {
        # "Cleanups the standalone mode and stop the execution.\nDon't remove 'GUI: Unregister Event', 'GUI: Cleanup Data' and 'Exit'."
        n74 = call <userlib>:"Enqueue.vi"("Queue in"=w194, "States"=string[] ["GUI: Unregister Event", "GUI: Cleanup Data", "Exit"], "Enqueue at Front?(F)"=TRUE, "error in (no error)"=w196) -> ("error out"=w197:errorcluster)  [unwired: 10 in, 1 out]
      }
      frame "--------------- GUI Mode-----------------" {
        # "Not used. category splitter"
      }
      frame "GUI: Initialize Data" {
        w220 = T6."Line Regulation Curve" ("Result Enum")
        w221 = T1."Station Setup" ("Tab Enum")
        w224 = string[][] []  # Test Results[][]
        w234 = T14 {"Frequency in Hz"=[], "Detected Vin_ac_pp in V"=[], "Detected Vout_ac_pp in V"=[], "PSRR in dB"=[], "Sample Rate in S/s"=[], "Record Length in S"=[]}  # Test Results
        # "Add the front panel controls terminal here and connect them to the bundle structure, So they will be available through data cluster in every case. If the controls and indicators are added to the 'Test Inputs' & 'Test Results' cluster then they are already available in the data cluster since they are typedefs."
        n75 = property on="Run" class="Bool (strict)"(error in=w228, "DisabledEnum"=T17."Enabled" ("Disabled")) -> (error out=w231:errorcluster)  [unwired: 1 in, 1 out]
        n76 = property on="Terminate" class="Bool (strict)"(error in=w231, "DisabledEnum"=T17."Disabled and Grayed Out" ("Disabled")) -> (error out=w227:errorcluster)  [unwired: 1 in, 1 out]
        n77 = property on="Progress" class="Slide (strict)"(error in=w227, "Visible"=FALSE) -> (error out=w226:errorcluster)  [unwired: 1 in, 1 out]
        n78 = local write "Tab Enum"(w221) -> ()
        n79 = local write "Tab Control"(w221) -> ()
        n80 = local write "Result Enum"(w220) -> ()
        n81 = local write "Result Tab"(w220) -> ()
        n82 = Bundle By Name(cluster=w233, "Test Pins"="Test Pins", "Test Inputs"="Test Inputs", "Test Results"=w234, "Test Results[][]"=w224, "Logger Folder Path"="DataLogPath") -> (w218:T16)
        n83 = control-ref of="Tab Enum"() -> (w214:refnum<vi>)
        n84 = control-ref of="Result Enum"() -> (w205:refnum<vi>)
        n85 = control-ref of="Customize Sweep Value"() -> (w207:refnum<vi>)
        n86 = control-ref of="Advanced Settings"() -> (w206:refnum<vi>)
        n87 = control-ref of="Take PSRR snapshot?"() -> (w204:refnum<vi>)
        n88 = control-ref of="SystemSetup"() -> (w216:refnum<vi>)
        n89 = control-ref of="Minimum Resolution Bandwidth (%)"() -> (w203:refnum<vi>)
        n90 = control-ref of="Sampling Rate Multiplier"() -> (w202:refnum<vi>)
        n91 = control-ref of="Input Voltage (V)"() -> (w213:refnum<vi>)
        n92 = control-ref of="Load Current (A)"() -> (w212:refnum<vi>)
        n93 = control-ref of="Pk-Pk Voltage (V)"() -> (w211:refnum<vi>)
        n94 = control-ref of="Maximum Frequency (Hz)"() -> (w208:refnum<vi>)
        n95 = control-ref of="Frequency (Hz)"() -> (w210:refnum<vi>)
        n96 = control-ref of="Minimum Frequency (Hz)"() -> (w209:refnum<vi>)
        n97 = Build Array(w216, w214, w213, w212, w211, w210, w209, w208, w207, w203, w202, w206, w205, w204) -> (w215:refnum<vi>[])
        n98 = Bundle By Name(cluster=w218, "UI Ctls"=w215) -> (w217:T16)
      }
      frame "GUI: Register Event" {
        # "Hidden in UI"
        # "Register for the events from caller."
        n99 = register-events(error in=w239, "Caller Events") -> (reference out=w236:refnum<event-registration>, error out=w237:errorcluster)  [unwired: 1 in]
      }
      frame "GUI: Unregister Event" {
        n100 = Unregister For Events(event registration refnum=w240, error in=w243) -> (error out=w241:errorcluster)
      }
      frame "GUI: Cleanup Data" {
        # "Cleanup the reference or other resources before exiting"
      }
      frame "GUI: Generate Frequency" {
        n101 = property on="Step Input" class="Clust (strict)"(error in=w257) -> (error out=w256:errorcluster, "Value"=w255:T19)  [unwired: 1 in, 1 out]
        n102 = Unbundle By Name(w255) -> ("Maximum Frequency Hz)"=w254:dbl, "Minimum Frequency (Hz)"=w253:dbl)
        n103 = call "Format Step Size Data.vi"("Max Frequency (Hz)"=w254, "Min Frequency (Hz)"=w253, "error in (no error)"=w256) -> ("Frequency[]"=w247:dbl[], "error out"=w250:errorcluster)  [unwired: 11 in]
        n104 = property on="Frequency (Hz)" class="Arr (strict)"(error in=w250, "Value"=w247) -> (error out=w252:errorcluster)  [unwired: 1 in, 1 out]
        n105 = Bundle By Name(cluster=w248, "Test Inputs.Frequency in Hz"=w247) -> (w249:T16)
        n106 = property on="Frequency in Hz" class="Arr (strict)"(error in=w252, "Value"=w247) -> (error out=w251:errorcluster)  [unwired: 1 in, 1 out]
      }
      frame "GUI: Update Measurement Table" {
        n107 = Unbundle By Name(w265) -> ("Test Results.Frequency in Hz"=w264:dbl[], "Test Results.Detected Vin_ac_pp in V"=w270:dbl[], "Test Results.Detected Vout_ac_pp in V"=w269:dbl[], "Test Results.PSRR in dB"=w268:dbl[], "Test Results.Sample Rate in S/s"=w263:dbl[], "Test Results.Record Length in S"=w262:dbl[])
        n108 = Build Array(w264, w270, w269, w268, w263, w262) -> (w267:dbl[][])
        n109 = for {
          tunnel: w267 -> [w275] mode=indexing
          tunnel: [w274] -> w260 mode=indexing
          tunnel: i16[] [0, 6, 6, 2, 2, 0] ("precision (6)") -> [w273] mode=indexing
          n110 = Number To Fractional String(number=w275, precision (6)=w273) -> (F-format string=w274:string[])  [unwired: 2 in]
        }
        n111 = Transpose 2D Array(2D array=w260) -> (transposed array=w259:string[][])
        "Measured Values" <- w259
        n112 = Bundle By Name(cluster=w265, "Test Results[][]"=w259) -> (w266:T16)
      }
      frame "GUI: Set Busy" {
        n113 = Unbundle By Name(w278) -> ("UI Ctls"=w282:refnum<vi>[])
        n114 = for {
          tunnel: [w287] -> w283 mode=indexing
          tunnel: w277 -> [w288]
          tunnel: w282 -> [w286] mode=indexing
          tunnel: T17."Disabled and Grayed Out" ("Disabled") -> [w285]
          n115 = property class="Ctl"(reference=w286, error in=w288, "DisabledEnum"=w285) -> (error out=w287:errorcluster)  [unwired: 1 out]
        }
        n116 = Merge Errors(w283) -> (w280:errorcluster)
        n117 = call "Defer Front Panel.vi"("Defer Front Panel?"=TRUE, "error in"=w280) -> ("error out"=w276:errorcluster)  [unwired: 13 in]
      }
      frame "GUI: Unset Busy" {
        n118 = Unbundle By Name(w291) -> ("UI Ctls"=w295:refnum<vi>[])
        n119 = for {
          tunnel: [w300] -> w296 mode=indexing
          tunnel: w290 -> [w301]
          tunnel: w295 -> [w299] mode=indexing
          tunnel: T17."Enabled" ("Disabled") -> [w298]
          n120 = property class="Ctl"(reference=w299, error in=w301, "DisabledEnum"=w298) -> (error out=w300:errorcluster)  [unwired: 1 out]
        }
        n121 = Merge Errors(w296) -> (w292:errorcluster)
        n122 = call "Defer Front Panel.vi"("Defer Front Panel?"=FALSE, "error in"=w292) -> ("error out"=w289:errorcluster)  [unwired: 13 in]
      }
      frame "GUI: Start Test" {
        n123 = property on="Run" class="Bool (strict)"(error in=w306, "DisabledEnum"=T17."Disabled and Grayed Out" ("Disabled")) -> (error out=w312:errorcluster)  [unwired: 1 in, 1 out]
        n124 = property on="Terminate" class="Bool (strict)"(error in=w312, "DisabledEnum"=T17."Enabled" ("Disabled")) -> (error out=w311:errorcluster)  [unwired: 1 in, 1 out]
        n125 = Unbundle By Name(w304) -> ("Test Inputs.Frequency in Hz"=w303:dbl[])
        n126 = Array Size(array=w303) -> (size(s)=w302:i32)
        n127 = property on="Progress" class="Slide (strict)"(error in=w311, "Visible"=TRUE, "Scale.Maximum"=w302, "Value"=0 ("Progress")) -> (error out=w307:errorcluster)  [unwired: 1 in, 1 out]
      }
      frame "GUI: Get Logger File Path" {
        n128 = Unbundle By Name(w315) -> ("Logger Folder Path"=w320:path)
        n129 = call <vilib>:"Check if File or Folder Exists.vi"("error in (no error)"=w321, "path"=w320) -> ("error out"=w318:errorcluster, "file or folder exists?"=w317:bool, "dup path"=w314:path)  [unwired: 7 in]
        n130 = case shown="True" w317 {
          tunnel: [w324 w333] -> w319
          tunnel: w318 -> [w324 w336]
          tunnel: w315 -> [w323 w340]
          tunnel: [w323 w339] -> w316
          tunnel: w314 -> [_ w335]
          frame False {
          }
          frame True {
            n131 = Strip Path(path=w335) -> (name=w327:string)  [unwired: 1 out]
            n132 = call "Get Unique Name.vi"() -> ("date"=w334:string, "Unique String"=w326:string)  [unwired: 14 in]
            n133 = Concatenate Strings(w327, w334) -> (w330:string)
            n134 = Concatenate Strings(w327, w326) -> (w325:string)
            n135 = Concatenate Strings(w330, "\\" ("string"), w325) -> (w337:string)
            n136 = Build Path(base path=w335, name or relative path=w337) -> (appended path=w332:path)
            n137 = call <vilib>:"Create Directory Recursive.vi"("error in (no error)"=w336, "directory"=w332) -> ("error out"=w333:errorcluster, "directory copy"=w329:path)  [unwired: 3 in, 1 out]
            n138 = Build Path(base path=w329, name or relative path=w325) -> (appended path=w328:path)
            n139 = Bundle By Name(cluster=w340, "Valid Logger path?"=TRUE, "Logger file path"=w328) -> (w339:T16)
          }
        }
      }
      frame "GUI: Log" {
        n140 = Unbundle By Name(w347) -> ("Valid Logger path?"=w341:bool, "Test Inputs"=w343:T7, "Test Results"=w344:T14, "Logger file path"=w342:path)
        n141 = case shown="True" w341 {
          tunnel: [w349 w354] -> w346
          tunnel: w345 -> [w349 w353]
          tunnel: w344 -> [_ w352]
          tunnel: w343 -> [_ w351]
          tunnel: w342 -> [_ w350]
          frame False {
          }
          frame True {
            n142 = call "Log Data.vi"("Test Inputs"=w351, "Test Results"=w352, "DataLogger File Path"=w350, "error in (no error)"=w353) -> ("error out"=w354:errorcluster)  [unwired: 11 in]
          }
        }
      }
      frame "GUI: PSRR Snapshot" {
        # "If you want to update more indicators in the front panel do it here. It is efficient to update the UI in one case rather than in several cases. Also, it is a good practice to store the results in the data cluster in an efficient format and then get the data from data cluster and update the UI, in that way we could have the front panel independent of how we manipulate the data."
        n143 = Unbundle By Name(w361) -> ("Test Inputs.Take PSRR snapshot?"=w358:bool, "Valid Logger path?"=w356:bool, "Logger file path"=w355:path)
        n144 = And(x=w358, y=w356) -> (x .and. y?=w357:bool)
        n145 = case shown="True" w357 {
          tunnel: w359 -> [w363 w369]
          tunnel: [w363 w371] -> w360
          tunnel: w355 -> [_ w364]
          frame False {
          }
          frame True {
            n146 = Path To String(path=w364) -> (string=w366:string)
            n147 = Concatenate Strings(w366, ".bmp" ("format string")) -> (w367:string)
            n148 = control-ref of="Frequency Vs PSRR"() -> (w370:refnum<vi>)
            n149 = String To Path(string=w367) -> (path=w365:path)
            n150 = invoke class="XYGraph (strict)" method="Export Image"(reference=w370, error in=w369, "FileType"=enum32{"BMP", "EPS", "EMF", "PICT"}."BMP" ("File Type"), "Target"=enum32{"File", "Clipboard"}."File", "Path"=w365) -> (error out=w371:errorcluster)  [unwired: 3 in, 7 out]
          }
        }
      }
      frame "GUI: End Test" {
        n151 = property on="Run" class="Bool (strict)"(error in=w376, "Value"=FALSE ("Run"), "DisabledEnum"=T17."Enabled" ("Disabled")) -> (error out=w381:errorcluster)  [unwired: 1 in, 1 out]
        n152 = property on="Terminate" class="Bool (strict)"(error in=w381, "DisabledEnum"=T17."Disabled and Grayed Out" ("Disabled")) -> (error out=w380:errorcluster)  [unwired: 1 in, 1 out]
        n153 = property on="Progress" class="Slide (strict)"(error in=w380, "Visible"=FALSE) -> (error out=w377:errorcluster)  [unwired: 1 in, 1 out]
      }
      frame "------------ TerminationMonitor -----------" {
        # "Not used. category splitter"
      }
      frame "TerminationMonitor: Start" {
        # "Termination Monitor monitors the execution of the caller. Use Termination Monitor Status to get the termination status. If the caller is terminating, stop the test procedure, cleanup and stop."
        n154 = Unbundle By Name(w389) -> ("Termination Monitor Info.Caller Information"=w388:T10)
        n155 = call <userlib>:"Termination Monitor Start.vi"("Caller Information"=w388, "error in (no error)"=w391) -> ("Termination Monitor Info out"=w387:T15, "error out"=w392:errorcluster)  [unwired: 12 in]
        n156 = Bundle By Name(cluster=w389, "Termination Monitor Info"=w387) -> (w390:T16)
      }
      frame "TerminationMonitor: Stop" {
        n157 = Unbundle By Name(w396) -> ("Termination Monitor Info"=w395:T15)
        n158 = call <userlib>:"Termination Monitor Stop.vi"("Status Info in"=w395, "error in (no error)"=w398) -> ("Status Info out"=w394:T15, "error out"=w399:errorcluster)  [unwired: 12 in]
        n159 = Bundle By Name(cluster=w396, "Termination Monitor Info"=w394) -> (w397:T16)
      }
      frame "------------ Automation Mode -----------" {
        # "Not used. category splitter"
      }
      frame "Test: Start" {
        # "Reinitialize/Reset/Update the data from the UI to the data cluster so that the data will be considered for the test procedure.\nReset the Test Results."
        n160 = local read "DataLogPath"() -> (w405:path)
        n161 = local read "Test Inputs"() -> (w404:T7)
        n162 = local read "Test Pins"() -> (w406:T13)
        n163 = property on="Run" class="Bool (strict)"(error in=w417, "DisabledEnum"=T17."Disabled and Grayed Out" ("Disabled")) -> (error out=w415:errorcluster)  [unwired: 1 in, 1 out]
        n164 = Bundle By Name(cluster=w420, "Test Pins"=w406, "Test Inputs"=w404, "Test Results"=T14 {"Frequency in Hz"=[], "Detected Vin_ac_pp in V"=[], "Detected Vout_ac_pp in V"=[], "PSRR in dB"=[], "Sample Rate in S/s"=[], "Record Length in S"=[]}, "Logger Folder Path"=w405) -> (w410:T16)
        n165 = property on="Terminate" class="Bool (strict)"(error in=w415, "DisabledEnum"=T17."Enabled" ("Disabled")) -> (error out=w412:errorcluster)  [unwired: 1 in, 1 out]
        n166 = Unbundle By Name(w410) -> ("Test Inputs.Frequency in Hz"=w409:dbl[])
        n167 = Array Size(array=w409) -> (size(s)=w408:i32)
        n168 = property on="Progress" class="Slide (strict)"(error in=w412, "Visible"=TRUE, "Scale.Maximum"=w408, "Value"=0 ("Progress")) -> (error out=w411:errorcluster)  [unwired: 1 in, 1 out]
      }
      frame "Test: Prepare DCPower" {
        # "Set Input voltage as initial voltage level\nSet first index of Load current as initial current"
        n169 = Unbundle By Name(w429) -> ("Test Pins.Set Load Current"=w423:string, "Test Inputs.Load Current in A"=w422:dbl, "Test Inputs.Advance Setting.Prepare.Load SMU Output Function"=w421:T9, "Test Pins.Set Input Voltage"=w426:string, "Test Inputs.Input Voltage in V"=w425:dbl)
        n170 = call "Prepare Source.vi"("Set Vin"=w426, "Initial Voltage Level (V)"=w425, "error in (no error)"=w427) -> ("error out"=w428:errorcluster)  [unwired: 12 in]
        n171 = call "Prepare Load.vi"("PinName"=w423, "Load Current Level (A)"=w422, "error in (no error)"=w428, "Load Output Function"=w421) -> ("error out"=w424:errorcluster)  [unwired: 11 in]
      }
      frame "Test: Prepare Scope" {
        w453 = 0 items=["AC", "DC", "Ground"] ("Vertical:Vertical Coupling")
        w447 = TRUE ("Vertical:Channel Enabled")
        # "Abort the acquisition"
        n172 = Unbundle By Name(w456) -> ("Test Pins.Measure Input Voltage"=w442:string, "Test Pins.Measure Output Voltage"=w449:string)
        n173 = call "Pin Name to Reference.vim"("Pin Name"=w449, "type"=refnum<k15> refnum ("instrument handle"), "error in (no error)"=w459) -> ("Reference"=w448:refnum<k15>, "Channel"=w444:string, "error out"=w451:errorcluster)  [unwired: 7 in, 3 out]
        n174 = call "Pin Name to Reference.vim"("Pin Name"=w442, "type"=refnum<k15> refnum ("instrument handle"), "error in (no error)"=w451) -> ("Reference"=w440:refnum<k15>, "Channel"=w445:string, "error out"=w450:errorcluster)  [unwired: 7 in, 3 out]
        n175 = call <instrlib>:"niScope Abort.vi"("instrument handle"=w440, "error in"=w450) -> ("instrument handle out"=w439:refnum<k15>, "error out"=w441:errorcluster)  [unwired: 12 in]
        n176 = property class="niScope"(reference=w439, error in=w441, "Active Channel"=w445, "Channel Enabled"=w447, "Vertical Coupling"=w453) -> (error out=w455:errorcluster)  [unwired: 1 out]
        n177 = property class="niScope"(reference=w448, error in=w455, "Active Channel"=w444, "Channel Enabled"=w447, "Vertical Coupling"=w453) -> (reference out=w437:refnum<k15>, error out=w454:errorcluster)
        n178 = property class="niScope"(reference=w437, error in=w454) -> (reference out=w436:refnum<k15>, error out=w438:errorcluster, "Enforce Realtime"=w435:bool, "Number of Records"=w434:i32, "Actual Sample Rate"=w433:dbl, "Reference Position"=w432:dbl, "Actual Record Length"=w431:i32)
        n179 = Concatenate Strings(w445, "," ("string"), w444) -> (w443:string)
        n180 = Bundle By Name(cluster=w456, "Scope Channels"=w443) -> (w457:T16)
        n181 = call <instrlib>:"niScope Configure Horizontal Timing.vi"("instrument handle"=w436, "number of records"=w434, "enforce realtime"=w435, "min sample rate"=w433, "reference position"=w432, "error in"=w438, "min record length"=w431) -> ("error out"=w458:errorcluster)  [unwired: 7 in, 1 out]
      }
      frame "Test: Set Input Voltage" {
        n182 = Unbundle By Name(w465) -> ("Test Pins.Set Input Voltage"=w463:string, "Test Inputs.Input Voltage in V"=w462:dbl)
        n183 = call "Set Source.vi"("Set Vin"=w463, "Vin in V"=w462, "error in (no error)"=w466) -> ("error out"=w464:errorcluster)  [unwired: 12 in]
      }
      frame "Test: Set Load Current" {
        n184 = Unbundle By Name(w472) -> ("Test Pins.Set Load Current"=w470:string, "Test Inputs.Load Current in A"=w469:dbl, "Test Inputs.Advance Setting.Prepare.Load SMU Output Function"=w468:T9)
        n185 = call "Set Load Current.vi"("PinName"=w470, "current level"=w469, "error in (no error)"=w473, "OutputFunction"=w468) -> ("error out"=w471:errorcluster)  [unwired: 11 in]
      }
      frame "Test: Sweep Over Frequency" {
        n186 = Unbundle By Name(w502) -> ("Termination Monitor Info"=w498:T15, "Test Inputs.Advance Setting.Stimulus and Measure.Search Tolerance (+/- % of Freq.)"=w475:dbl, "Test Inputs.Frequency in Hz"=w490:dbl[], "Scope Channels"=w486:string, "Test Inputs.Advance Setting.Stimulus and Measure.Loop Delay"=w477:u32, "Test Inputs.Advance Setting.Stimulus and Measure.Autoset Sampling Rate?"=w476:bool, "Test Inputs.Resolution bandwidth in %"=w479:dbl, "Test Inputs.Sampling Rate multiplier"=w478:dbl, "Test Inputs.FGen Peak-Peak Voltage in V"=w482:dbl, "Test Pins.Set Frequency"=w487:string, "Test Pins.Measure Input Voltage"=w488:string)
        n187 = call "Pin Name to Reference.vim"("Pin Name"=w488, "type"=refnum<k15> refnum ("instrument handle"), "error in (no error)"=w497) -> ("Reference"=w492:refnum<k15>, "error out"=w494:errorcluster)  [unwired: 7 in, 4 out]
        n188 = call "Pin Name to Reference.vim"("Pin Name"=w487, "type"=refnum<k15> refnum ("instrument handle"), "error in (no error)"=w494) -> ("Reference"=w493:refnum<k15>, "error out"=w489:errorcluster)  [unwired: 7 in, 4 out]
        n189 = for {
          shift-right: [w521] -> w499
          shift-left: w489 -> [w542]
          shift-right: [w544] -> w491
          shift-left: w498 -> [w545]
          tunnel: w490 -> [w513] mode=indexing
          tunnel: w493 -> [w541]
          tunnel: w492 -> [w514]
          tunnel: w486 -> [w536]
          tunnel: [w513] -> w485 mode=indexing
          tunnel: [w540] -> w484 mode=indexing
          tunnel: [w539] -> w483 mode=indexing
          tunnel: w482 -> [w538]
          tunnel: [w519] -> w480 mode=indexing
          tunnel: [w523] -> w481 mode=indexing
          tunnel: w479 -> [w512]
          tunnel: w478 -> [w511]
          tunnel: w477 -> [w505]
          tunnel: w476 -> [w504]
          tunnel: w475 -> [w503]
          i -> [w543]
          stop <- w518 stop-if-true
          w526 = T20 0 items=["Sine", "Square", "Triangle", "Ramp Up", "Ramp Down", "DC", "Noise", "User"] ("Waveform")
          w527 = T21 0 items=["Standard Function", "Frequency List", "Arbitrary Waveform", "Arbitrary Sequence", "Script"] ("output mode")
          n190 = call <instrlib>:"niFgen Abort Generation.vi"("error in (no error)"=w542, "Instrument Handle"=w541) -> ("error out"=w531:errorcluster, "Instrument Handle Out"=w530:refnum<k15>)  [unwired: 8 in]
          n191 = call <instrlib>:"niFgen Configure Output Mode.vi"("error in (no error)"=w531, "Output Mode (default: 0=Standard Function)"=w527, "Instrument Handle"=w530) -> ("error out"=w534:errorcluster, "Instrument Handle Out"=w535:refnum<k15>)  [unwired: 6 in]
          n192 = call <instrlib>:"niFgen Configure Standard Waveform.vi"("Instrument Handle"=w535, "Waveform"=w526, "Frequency"=w513, "Amplitude"=w538, "error in (no error)"=w534, "DC Offset"=0.0) -> ("Instrument Handle Out"=w532:refnum<k15>, "error out"=w533:errorcluster)  [unwired: 8 in]
          n193 = call <instrlib>:"niFgen Output Enable.vi"("error in (no error)"=w533, "Output Enable (default: True)"=TRUE ("output enable"), "Instrument Handle"=w532) -> ("error out"=w529:errorcluster, "Instrument Handle Out"=w528:refnum<k15>)  [unwired: 7 in]
          n194 = call <instrlib>:"niFgen Initiate Generation.vi"("error in (no error)"=w529, "Instrument Handle"=w528) -> ("error out"=w515:errorcluster)  [unwired: 8 in, 1 out]
          n195 = call "Check Sampling Rate and Record Length Support.vi"("Scope Reference"=w514, "Autoset Sampling Rate?"=w504, "Frequency Sweep"=w513, "Resolution Bandwidth(%)"=w512, "Sampling Rate Multiplier"=w511, "error in"=w515) -> ("Scope Reference Out"=w520:refnum<k15>, "Minimum Sampling Rate"=w509:dbl, "Minimum Record Length"=w508:i32, "Parameter Supported?"=w516:bool, "Maximum Record length"=w506:i32, "Maximum Sampling Rate"=w507:dbl, "error out"=w510:errorcluster)  [unwired: 3 in]
          n196 = case shown="True" w516 {
            tunnel: w513 -> [_ w579]
            tunnel: [_ w578] -> w540
            tunnel: [_ w577] -> w539
            tunnel: w505 -> [_ w575]
            tunnel: w536 -> [_ w574]
            tunnel: [_ w560] -> w523
            tunnel: [w551 w570] -> w522
            tunnel: w503 -> [_ w567]
            tunnel: w510 -> [w550 w565]
            tunnel: w520 -> [_ w564]
            tunnel: [_ w559] -> w519
            tunnel: [TRUE FALSE] -> w517
            tunnel: w509 -> [w549 w563]
            tunnel: w508 -> [w548 w562]
            tunnel: w507 -> [w547 _]
            tunnel: w506 -> [w546 _]
            frame False {
              # "Throw error and stop Acquisition, Measure"
              n197 = call "Error 6002.vi"("Requested Sampling Rate"=w549, "Requested Record Length"=w548, "Maximum Sampling Rate"=w547, "Maximum Record Length"=w546, "error in (no error)"=w550) -> ("error out"=w551:errorcluster)  [unwired: 10 in]
            }
            frame True {
              # "Sample Rate and Record length supported"
              n198 = call "Configure Horizontal Timing.vi"("Scope Reference"=w564, "Minimum Sampling Rate (S/s)"=w563, "Record Length"=w562, "error in"=w565) -> ("Scope Reference Out"=w556:refnum<k15>, "error out"=w554:errorcluster)  [unwired: 10 in]
              n199 = call "Limit Record Length.vi"("Scope Reference"=w556, "error in (no error)"=w554) -> ("Scope Reference Out"=w555:refnum<k15>, "error out"=w553:errorcluster)  [unwired: 12 in]
              n200 = property class="niScope"(reference=w555, error in=w553) -> (reference out=w558:refnum<k15>, error out=w557:errorcluster, "Actual Record Length"=w561:i32, "Actual Sample Rate"=w559:dbl)
              n201 = call <instrlib>:"niScope Initiate Acquisition.vi"("instrument handle"=w558, "error in"=w557) -> ("instrument handle out"=w571:refnum<k15>, "error out"=w576:errorcluster)  [unwired: 12 in]
              n202 = To Double Precision Float(number=w561) -> (double precision float=w560:dbl)
              n203 = call "Stall Data Flow.vim"("value in"=w576, "milliseconds to wait"=w575) -> ("value out"=w572:errorcluster)  [unwired: 1 out]
              n204 = call "Measure Voltage Waveform.vi"("Scope Reference"=w571, "Scope Channels"=w574, "Record Length"=w560, "Actual Sample Rate"=w559, "error in (no error)"=w572) -> ("Input Waveform"=w569:T22, "Output Waveform"=w568:T22, "error out"=w573:errorcluster)  [unwired: 8 in]
              n205 = call "Extract Peak-Peak Voltage.vi"("Input Waveform"=w569, "Frequency (Hz)"=w579, "Search %"=w567, "Output Waveform"=w568, "Actual Sample Rate"=w559, "error in (no error)"=w573) -> ("Detected Output Voltage"=w578:dbl, "Detected Input Voltage"=w577:dbl, "error out"=w570:errorcluster)  [unwired: 7 in]
            }
          }
          n206 = call <userlib>:"Termination Monitor Status.vi"("Termination Monitor Info in"=w545, "error in (no error)"=w522) -> ("Termination Monitor Info out"=w544:T15, "Terminating?"=w537:bool, "error out"=w521:errorcluster)  [unwired: 11 in]
          n207 = Or(x=w537, y=w517) -> (x .or. y?=w518:bool)
          "Progress" <- w543
        }
        n208 = Bundle By Name(cluster=w502, "Termination Monitor Info"=w491, "Test Results.Frequency in Hz"=w485, "Test Results.Detected Vout_ac_pp in V"=w484, "Test Results.Detected Vin_ac_pp in V"=w483, "Test Results.Record Length in S"=w481, "Test Results.Sample Rate in S/s"=w480) -> (w501:T16)
      }
      frame "Test: Cleanup DCPower" {
        n209 = Unbundle By Name(w597) -> ("Test Pins.Set Load Current"=w592:string, "Test Pins.Set Input Voltage"=w594:string)
        n210 = call "Pin Name to Reference.vim"("Pin Name"=w594, "type"=refnum<k15> refnum ("instrument handle"), "error in (no error)"=w595) -> ("Reference"=w588:refnum<k15>, "error out"=w589:errorcluster)  [unwired: 7 in, 4 out]
        n211 = call <instrlib>:"niDCPower Configure Output Enabled.vi"("error in (no error)"=w589, "output enabled"=FALSE, "instrument handle"=w588) -> ("error out"=w586:errorcluster, "instrument handle out"=w587:refnum<k15>)  [unwired: 7 in]
        n212 = call <instrlib>:"niDCPower Abort With Channels.vi"("error in (no error)"=w586, "instrument handle"=w587) -> ("error out"=w585:errorcluster)  [unwired: 8 in, 1 out]
        n213 = call "Pin Name to Reference.vim"("Pin Name"=w592, "type"=refnum<k15> refnum ("instrument handle"), "error in (no error)"=w585) -> ("Reference"=w583:refnum<k15>, "error out"=w584:errorcluster)  [unwired: 7 in, 4 out]
        n214 = call <instrlib>:"niDCPower Configure Output Enabled.vi"("error in (no error)"=w584, "output enabled"=FALSE, "instrument handle"=w583) -> ("error out"=w582:errorcluster, "instrument handle out"=w581:refnum<k15>)  [unwired: 7 in]
        n215 = call <instrlib>:"niDCPower Abort With Channels.vi"("error in (no error)"=w582, "instrument handle"=w581) -> ("error out"=w580:errorcluster)  [unwired: 8 in, 1 out]
      }
      frame "Test: Cleanup Fgen" {
        n216 = Unbundle By Name(w608) -> ("Test Pins.Set Frequency"=w605:string)
        n217 = call "Pin Name to Reference.vim"("Pin Name"=w605, "type"=refnum<k15> refnum ("instrument handle"), "error in (no error)"=w606) -> ("Reference"=w601:refnum<k15>, "error out"=w602:errorcluster)  [unwired: 7 in, 4 out]
        n218 = call <instrlib>:"niFgen Output Enable.vi"("error in (no error)"=w602, "Output Enable (default: True)"=FALSE, "Instrument Handle"=w601) -> ("error out"=w603:errorcluster, "Instrument Handle Out"=w600:refnum<k15>)  [unwired: 7 in]
        n219 = call <instrlib>:"niFgen Abort Generation.vi"("error in (no error)"=w603, "Instrument Handle"=w600) -> ("error out"=w599:errorcluster)  [unwired: 8 in, 1 out]
      }
      frame "Test: Cleanup Scope" {
        w610 = FALSE
        n220 = Unbundle By Name(w626) -> ("Test Pins.Measure Output Voltage"=w619:string, "Test Pins.Measure Input Voltage"=w623:string)
        n221 = call "Pin Name to Reference.vim"("Pin Name"=w623, "type"=refnum<k15> refnum ("instrument handle"), "error in (no error)"=w624) -> ("Reference"=w617:refnum<k15>, "Channel"=w614:string, "error out"=w621:errorcluster)  [unwired: 7 in, 3 out]
        n222 = property class="niScope"(reference=w617, error in=w621, "Active Channel"=w614, "Channel Enabled"=w610) -> (error out=w618:errorcluster)  [unwired: 1 out]
        n223 = call "Pin Name to Reference.vim"("Pin Name"=w619, "type"=refnum<k15> refnum ("instrument handle"), "error in (no error)"=w618) -> ("Reference"=w615:refnum<k15>, "Channel"=w613:string, "error out"=w620:errorcluster)  [unwired: 7 in, 3 out]
        n224 = property class="niScope"(reference=w615, error in=w620, "Active Channel"=w613, "Channel Enabled"=w610) -> (reference out=w611:refnum<k15>, error out=w616:errorcluster)
        n225 = call <instrlib>:"niScope Abort.vi"("instrument handle"=w611, "error in"=w616) -> ("error out"=w612:errorcluster)  [unwired: 12 in, 1 out]
      }
      frame "Test: Calculate PSRR" {
        n226 = Unbundle By Name(w634) -> ("Test Results.Detected Vin_ac_pp in V"=w633:dbl[], "Test Results.Detected Vout_ac_pp in V"=w632:dbl[])
        n227 = Divide(x=w633, y=w632) -> (x/y=w628:dbl[])
        n228 = Logarithm Base 10(1:w628) -> (0:w629:dbl[])
        n229 = Multiply(x=20.0, y=w629) -> (x*y=w631:dbl[])
        n230 = Bundle By Name(cluster=w634, "Test Results.PSRR in dB"=w631) -> (w635:T16)
      }
      frame "Test: Update UI" {
        # "If you want to update more indicators in the front panel do it here. It is efficient to update the UI in one case rather than in several cases. Also, it is a good practice to store the results in the data cluster in an efficient format and then get the data from data cluster and update the UI, in that way we could have the front panel independent of how we manipulate the data."
        n231 = Unbundle By Name(w644) -> ("Test Results.Frequency in Hz"=w642:dbl[], "Test Results"=w641:T14)
        "Test Results" <- w641
        n232 = Unbundle By Name(w641) -> ("PSRR in dB"=w640:dbl[])
        n233 = Bundle("Frequency in Hz"=w642, "PSRR in dB"=w640) -> (→"Frequency Vs PSRR":T23)  [unwired: 1 in]
      }
      frame "Test: End" {
        # "End of the Test Procedure. Do cleanup of resources or references."
        n234 = property on="Run" class="Bool (strict)"(error in=w650, "Value"=FALSE ("Run"), "DisabledEnum"=T17."Enabled" ("Disabled")) -> (error out=w653:errorcluster)  [unwired: 1 in, 1 out]
        n235 = property on="Terminate" class="Bool (strict)"(error in=w653, "DisabledEnum"=T17."Disabled and Grayed Out" ("Disabled")) -> (error out=w648:errorcluster)  [unwired: 1 in, 1 out]
        n236 = property on="Progress" class="Slide (strict)"(error in=w648, "Visible"=FALSE, "Value"=0 ("Progress")) -> (error out=w647:errorcluster)  [unwired: 1 in, 1 out]
      }
      frame "---------------------Misc-----------------------" {
      }
      frame "Error" {
        # "Handle the error and make sure to clear the error."
        n237 = Unbundle By Name(w662) -> ("Termination Monitor Info.Caller Information.Mode"=w661:T11)
        n238 = case shown="\"MeasurementSuite\"" w661 {
          tunnel: w665 -> [w669 w674 w676]
          tunnel: [w667 w671 w675] -> w663
          tunnel: [_ TRUE _] -> w660
          tunnel: w659 -> [_ w672 _]
          frame "Standalone" {
            w666 = T24 2 items=["no dialog", "OK message", "continue or stop message", "OK message + warnings", "continue/stop + warnings"] ("type of dialog (OK msg:1)")
            n239 = call <vilib>:"General Error Handler.vi"("type of dialog (OK msg:1)"=w666, "error in (no error)"=w669) -> ("error out"=w668:errorcluster)  [unwired: 9 in, 4 out]
            n240 = call <vilib>:"Clear Errors.vi"("error in (no error)"=w668) -> ("error out"=w667:errorcluster)  [unwired: 5 in, 1 out]
          }
          frame "Automation" {
            n241 = call <userlib>:"Release.vi"("Queue in"=w672) -> ("Error Out"=w670:errorcluster)  [unwired: 14 in]
            n242 = Merge Errors(w674, w670) -> (w671:errorcluster)
          }
          frame "MeasurementSuite" {
            n243 = property on="ErrorOccured" class="Clust (strict)"("Val(Sgnl)"=w676) -> (error out=w675:errorcluster)  [unwired: 2 in, 1 out]
          }
        }
      }
      frame "Exit" {
        # "Last case called before stopping the execution. \nError occured in this state will not be captured by Error state."
        n244 = call <userlib>:"Release.vi"("Queue in"=w682, "Error In"=w683) -> ("Error Out"=w678:errorcluster)  [unwired: 13 in]
        n245 = property on="Progress" class="Slide (strict)"(error in=w678, "Visible"=TRUE) -> (error out=w677:errorcluster)  [unwired: 1 in, 1 out]
      }
    }
  }
  "error out" <- w4
  "Header" <- "PSRR" ("Header")
